vi "Project Wizard.vi"() -> ()   [LabVIEW 2021]
uses:
  Control/Tab Control.ctl
  Control/Available Sample List.ctl
  Control/Available List Item.ctl
  <vilib>/myRIO/Common/Instrument Driver Framework/Utilities/xctls/myRIO Choice Button/myRIO Choice Button.xctl
  Control/Shared Values.ctl
  Control/Item List.ctl
  Control/Item Info.ctl
  Control/Answers.ctl
  Control/Question.ctl
  Control/Answer.ctl
  Control/FP Values.ctl
  Control/Navigation Control.ctl
  Control/States.ctl
  <resource>/dialog/NewProjectWizard/SpecPage/Base/BaseSpecPage.lvclass
  <vilib>/event_ctls.llb/eventvkey.ctl
  <resource>/dialog/NewProjectWizard/MetaDataObj/MetaDataObj.lvclass/MetaDataObj.ctl
  <vilib>/Utility/miscctls.llb/LVRectTypeDef.ctl
  <resource>/dialog/NewProjectWizard/Spec Page Interface.ctl
  <resource>/dialog/NewProjectWizard/MetaDataObj/Accessors/Read Project Root.vi
  <resource>/dialog/NewProjectWizard/MetaDataObj/Accessors/Read File Prefix.vi
  <resource>/dialog/NewProjectWizard/MetaDataObj/Accessors/Read Project Name.vi
  <resource>/dialog/NewProjectWizard/MetaDataObj/Accessors/Read Overlay Pixmap.vi
  <resource>/dialog/NewProjectWizard/MetaDataObj/Accessors/Write Project Root.vi
  <vilib>/Utility/cursorutil.llb/Set Cursor (Icon Pict).vi
  <vilib>/Utility/xml.llb/Read From XML File(string).vi
  <vilib>/Platform/browser.llb/Open URL in Default Browser (path).vi
  <resource>/dialog/NewProjectWizard/MetaDataObj/Accessors/Read Custom VI Path.vi
  <resource>/dialog/NewProjectWizard/MetaDataObj/Accessors/Read Project Path.vi
  SubVI/Wizard Global.vi
  <resource>/dialog/NewProjectWizard/MetaDataObj/Accessors/Read Title.vi
  <resource>/dialog/NewProjectWizard/MetaDataObj/MetaDataObj.lvclass
  <vilib>/LabVIEW Icon API/lv_icon/Classes/Icon/Icon.lvclass
  <resource>/dialog/NewProjectWizard/Loading Project Info/NI_NPW_Loading Project Info.lvlib
  <resource>/dialog/NewProjectWizard/Filters/NI_NPW_Filters.lvlib
  <resource>/dialog/lvconfig.llb/LV Config Read Pathlist.vi
  <resource>/dialog/NewProjectWizard/MetaDataObj/Convert To Child Class.vi
  <resource>/dialog/NewProjectWizard/Init Spec Page.vi
  <resource>/dialog/NewProjectWizard/Build Error String.vi
  SubVI/Tab Key Process.vi
  <resource>/dialog/NewProjectWizard/ValidateFilePath.vi
  <resource>/dialog/lvconfig.llb/LV Config Write Pathlist.vi
  <resource>/dialog/NewProjectWizard/Project Copying/CreateUserProject.vi
  <resource>/dialog/NewProjectWizard/Project Copying/NI_NPW_Project Copying.lvlib
  <vilib>/Utility/cursorutil.llb/Set Busy.vi
  <resource>/dialog/NewProjectWizard/Defer Panel Updates.vi
panel:
  in  "Tab Control":T1
  in  "Choice 2":bool(xcontrol)
  in  "Choice 1":bool(xcontrol)
  out "Question":string="What's your task?"
  out "Recommended sample":string
  out "Recommend":string="Recommended sample project: "
  out "Description":string
  out "Sample Pic 2":picture caption="Template Pic"
  in  "More Information":string="More Information"
  in  "Scrollbar":i32(c297)
  in  "Sample Project":T2={"List Item"={"Name"="", "Description"="", "More Info"="More Information"}, "List Item 2"={"Name"="", "Description"="", "More Info"="More Information"}, "List Item 3"={"Name"="", "Description"="", "More Info"="More Information"}, "List Item 4"={"Name"="", "Description"="", "More Info"="More Information"}, "List Item 5"={"Name"="", "Description"="", "More Info"="More Information"}}
  in  "Sample Highlight":picture
  in  "Category:":string(tree)="Connection 2"
  out "Sample Pic":picture
  out "Error Messages":string
  in  "Cancel":bool
  in  "Next":bool
  in  "Back":bool
  # "Sample Project:"
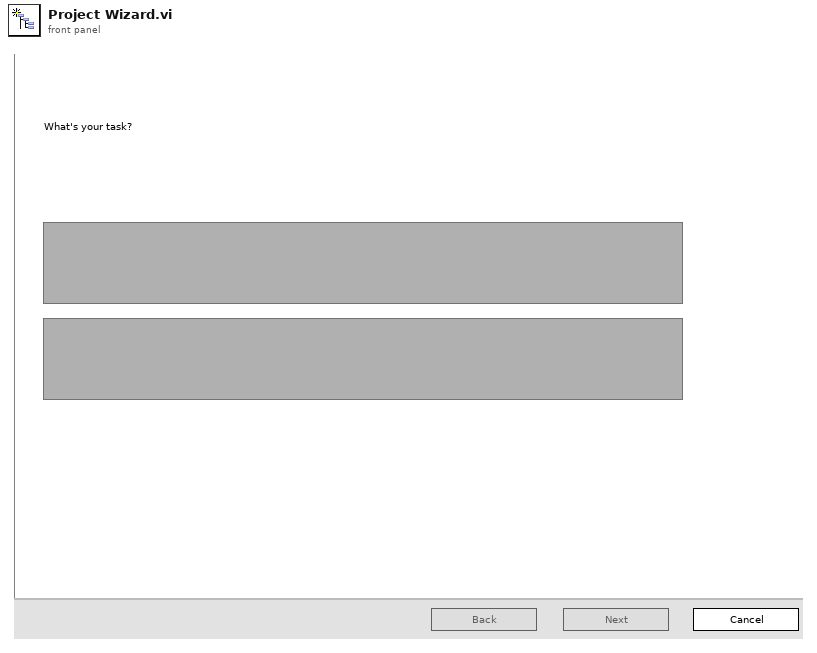
[diagram p1: front panel]
types:
  T1 = typedef "Tab Control.ctl" = enum32{"Start Page", "Recommend Sample", "Select Sample", "Configure Project"}
  T2 = typedef "Available Sample List.ctl" = cluster{"List Item":T3, "List Item 2":T3, "List Item 3":T3, "List Item 4":T3, "List Item 5":T3}
  T3 = typedef "Available List Item.ctl" = cluster{"Name":string, "Description":string, "More Info":string}
  T4 = typedef "States.ctl" = enum16{"Idle", "Initialize", "Parse Config Files", "Update Title", "Update Navigation", "Update Tab", "Load Question", "Load All Samples", "Update Sample Description", "Load Available Samples", "Cancel", "More Information", "Create Project", "Copy Project", "Update Warning", "Update Available Samples", "Select Available Sample", "Load Start Choice", "Show Recommended Sample", "Init Spec Page", "Insert Spec Page", "Stop Spec Page", "Set Control Font", "Focus Previous Selection"}
  T5 = typedef "FP Values.ctl" = cluster{"Title Index":i32, "Navigation Status":T6, "Selected Question":i32, "Selected Sample":i32, "Warning":string, "Sample Filter":string, "Available Items":T3[], "Scrollbar Value":i32, "Question":string, "Result":string, "Answers":T7, "Show Guidance":bool, "Tab Control":T1, "Previous Selection":T7}
  T6 = typedef "Navigation Control.ctl" = enum16{"Back Disable&Next", "Back Enable&Finish Disable", "Back Enable&Next", "Back Diable&Finish", "Back Enable&Finish", "Back Enable&Next Disable", "Back Disable&Next Disable"}
  T7 = typedef "Answers.ctl" = enum16{"Choice 1", "Choice 2"}
  T8 = typedef "Shared Values.ctl" = cluster{"Item List":T9, "Have Next Page":bool, "Next Page\n Index":i32, "User changed folder":bool, "Question Selection":i32[], "Selected Choices":T7[], "Sample Item Names":string[], "Displayed Available Sample":T3[], "Question List":T11[], "CurPage Ctrl #1":refnum<vi>, "CurPage Ctrl #n":refnum<vi>, "User Project":refnum<vi>, "Spec Page Reference":refnum<vi>, "Current Choice Index":i32}
  T9 = typedef "Item List.ctl" = T10[]
  T10 = typedef "Item Info.ctl" = cluster{"Tag Name":string, "Text":string, "Parent Tag":string, "Children Tags":string[], "Description":string, "Pic Name":string, "Is Root":bool, "Is Leaf":bool, "Sample Folder Name":string, "Documentation Name":string}
  T11 = typedef "Question.ctl" = cluster{"Text":string, "Choice 1":T12, "Choice 2":T12}
  T12 = typedef "Answer.ctl" = cluster{"Text":string, "ReachSample":bool, "Sample":string, "NextQuestion":i32}
  T13 = typedef "eventvkey.ctl" = enum16{"ASCII", "Enter", "Return", "Shift", "Ctrl", "Alt", "Cmd", "Opt", "Caps", "NumLock", "Clear", "Break", "Up", "Down", "Left", "Right", "Insert", "Delete", "Home", "End", "PageUp", "PageDown", "Escape", "Help", "Pause", "ScrollLock", "F1", "F2", "F3", "F4", "F5", "F6", "F7", "F8", "F9", "F10", "F11", "F12", "F13", "F14", "F15", "F16", "F17", "F18", "F19", "F20", "F21", "F22", "F23", "F24", "Play", "VolumeUp", "VolumeDown", "Mute", "Two Byte Char"}
  T14 = typedef "LVRectTypeDef.ctl" = cluster{"Left":i16, "Top":i16, "Right":i16, "Bottom":i16}
  T15 = enum8{"Enabled", "Disabled", "Disabled and Grayed Out"}
  T16 = typedef "LVPositionTypeDef.ctl" = cluster{"Left":i32, "Top":i32}
  T17 = typedef "Spec Page Interface.ctl" = cluster{"\"Tab Forward To\" Refnum":refnum<vi>, "\"Tab Backward To\" Refnum":refnum<vi>, "Errors":refnum<user-event>, "Quit":refnum<user-event>}
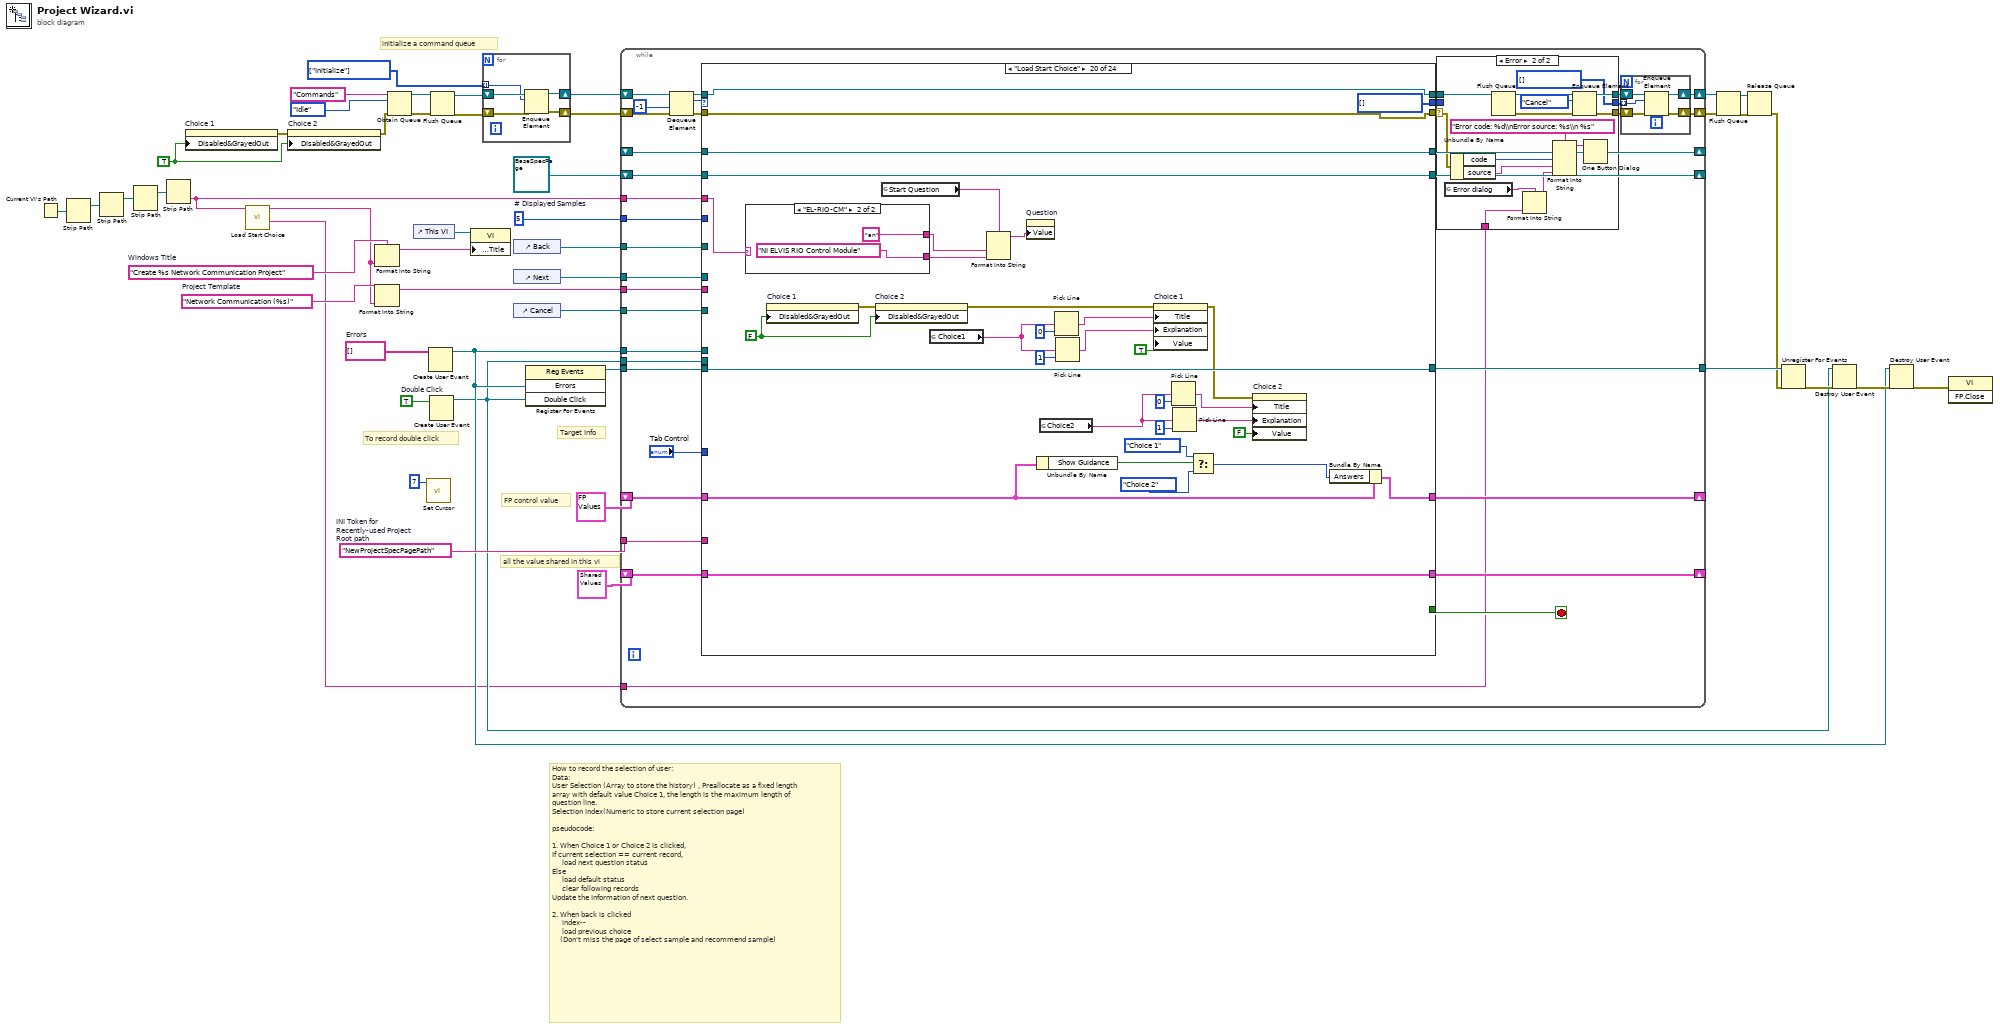
[diagram p0: block diagram]
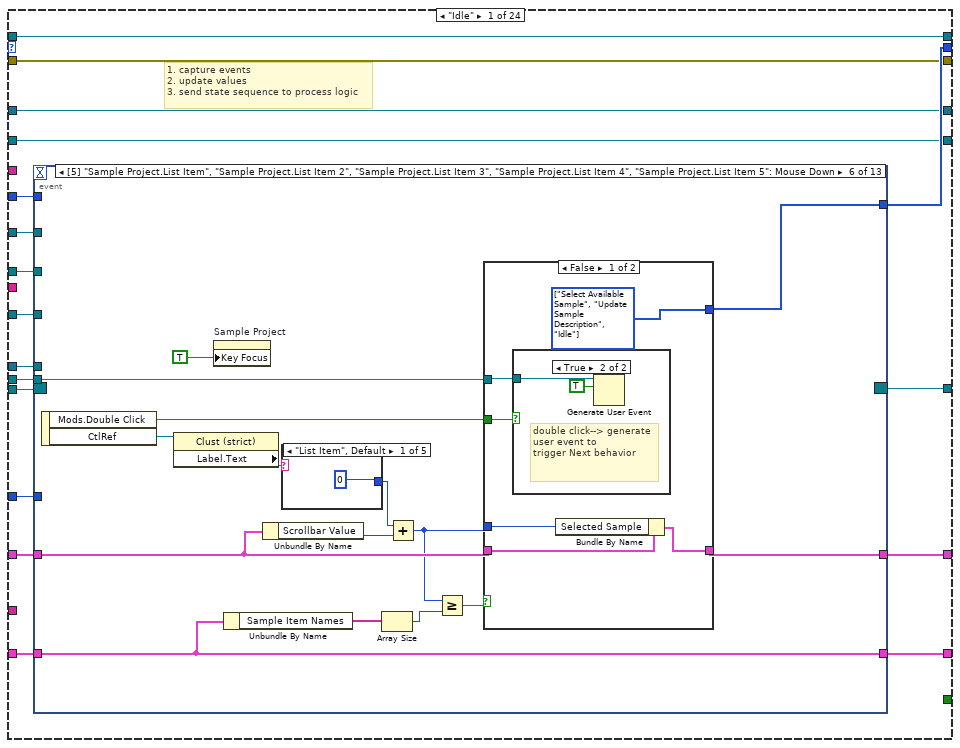
[diagram p3: hidden frame]
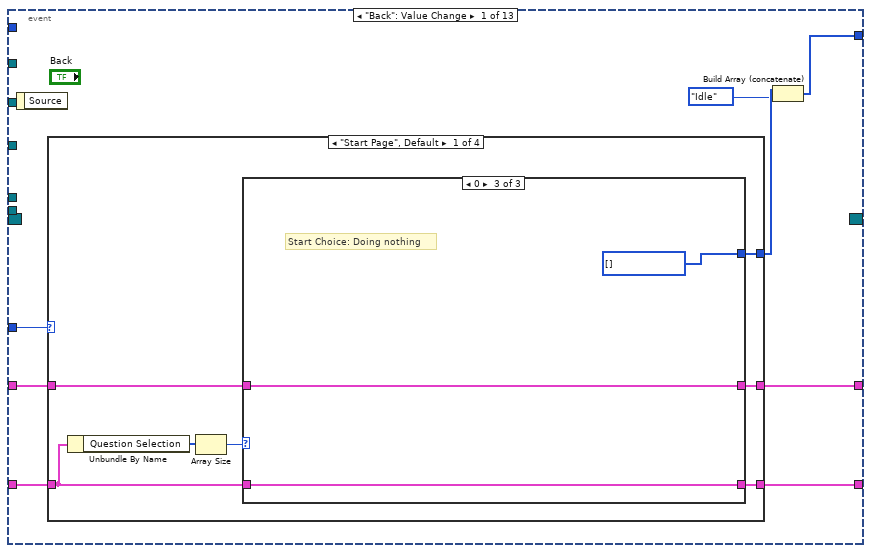
[diagram p4: hidden frame]
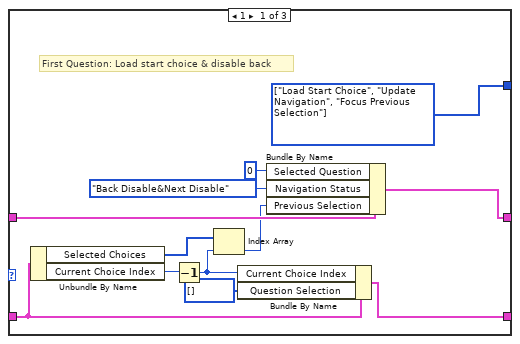
[diagram p5: hidden frame]
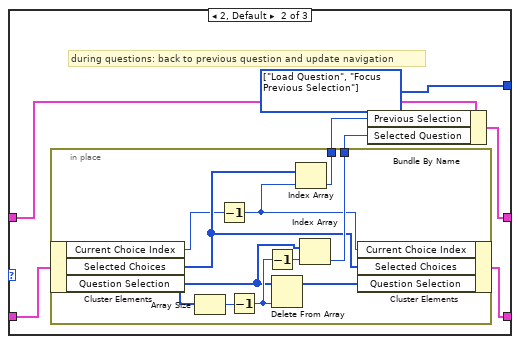
[diagram p6: hidden frame]
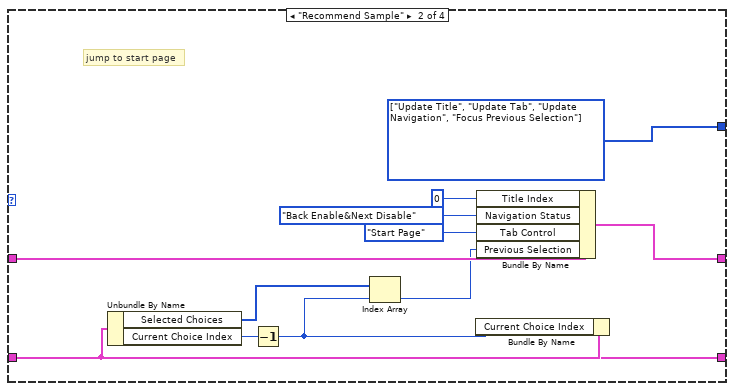
[diagram p7: hidden frame]
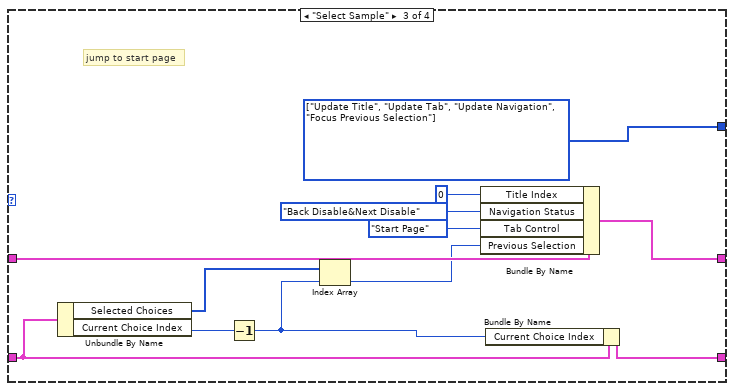
[diagram p8: hidden frame]
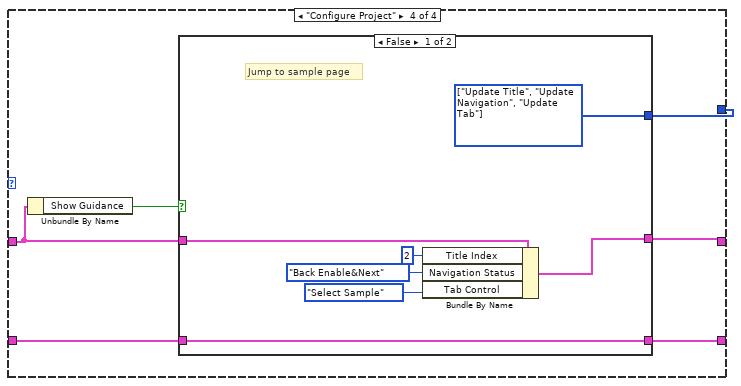
[diagram p9: hidden frame]
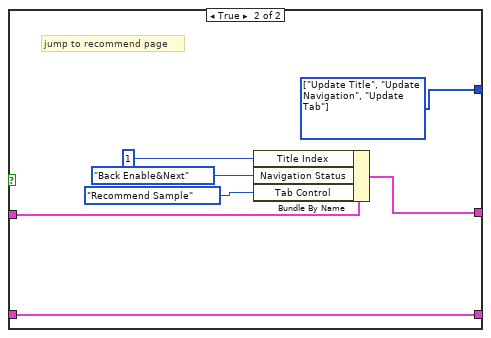
[diagram p10: hidden frame]
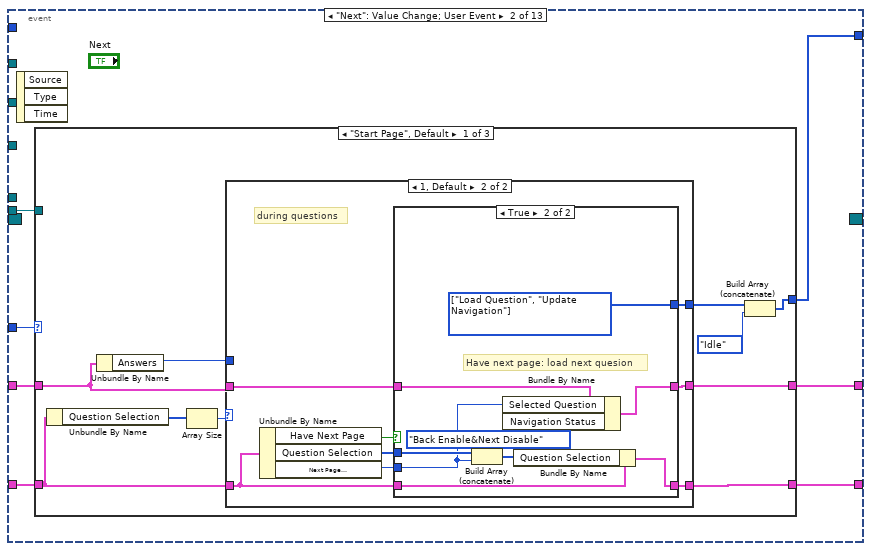
[diagram p11: hidden frame]
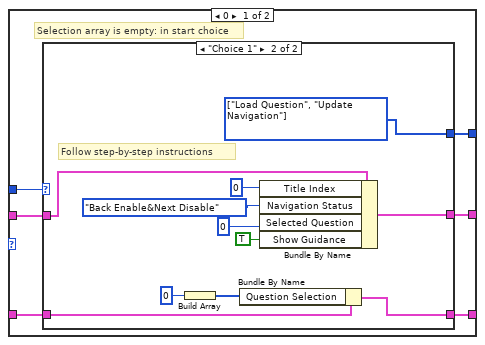
[diagram p12: hidden frame]
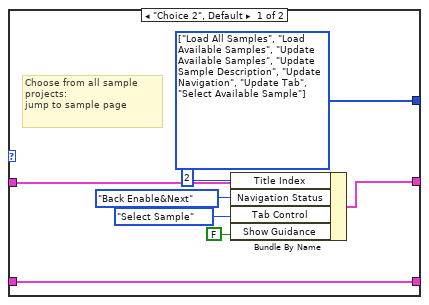
[diagram p13: hidden frame]
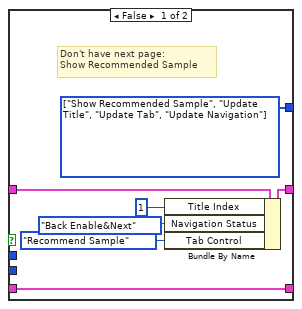
[diagram p14: hidden frame]
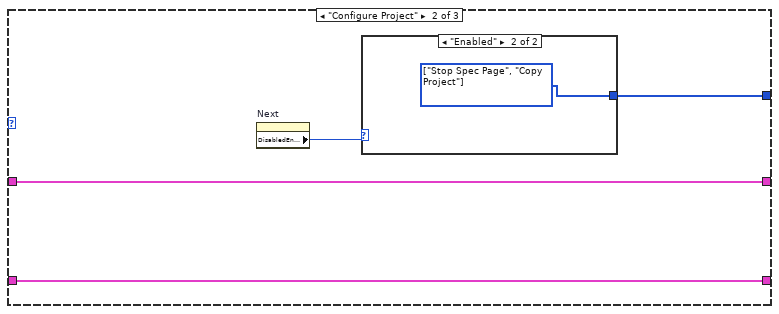
[diagram p15: hidden frame]
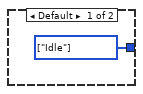
[diagram p16: hidden frame]
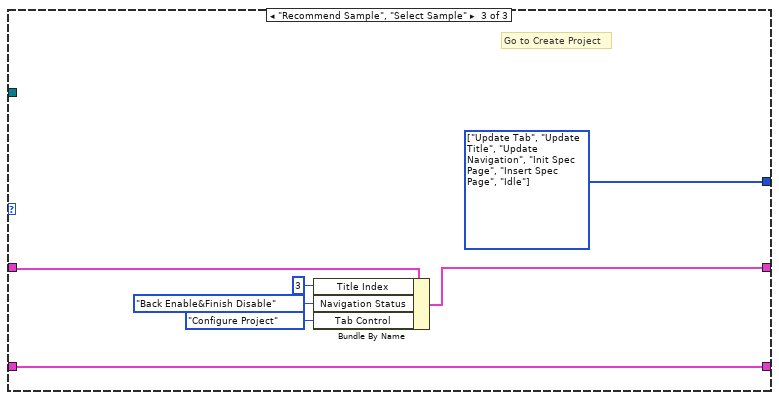
[diagram p17: hidden frame]
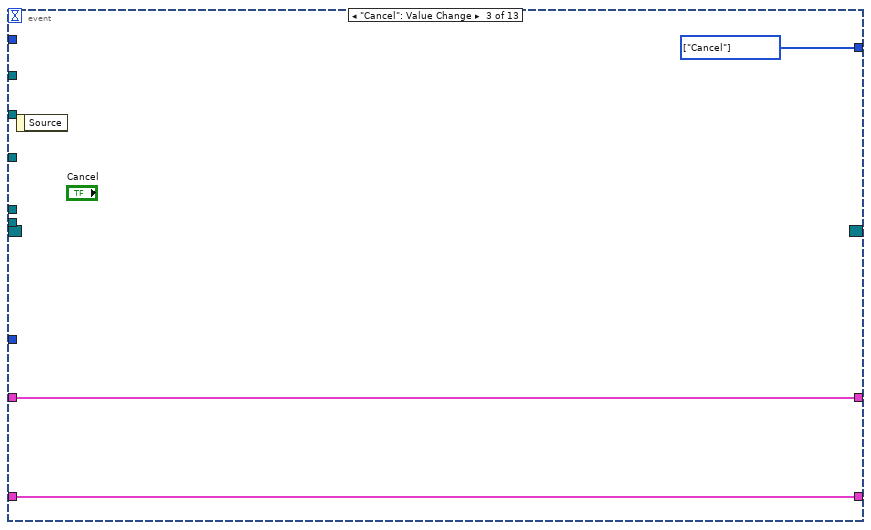
[diagram p18: hidden frame]
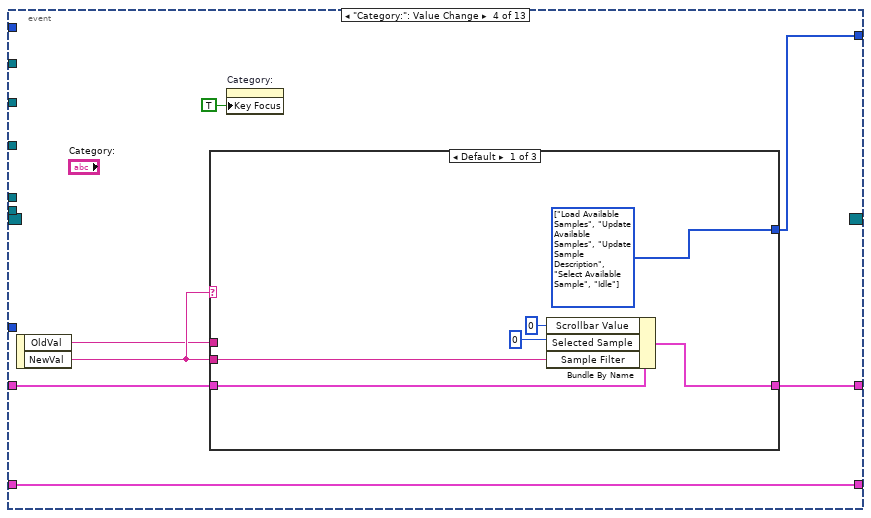
[diagram p19: hidden frame]
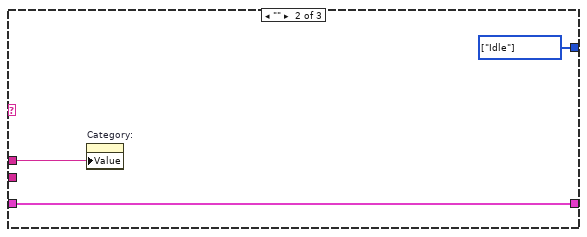
[diagram p20: hidden frame]
diagram:
  w11 = "Create %s Network Communication Project"  # Windows Title
  w18 = TRUE ("Disabled&GrayedOut")
  w25 = TRUE  # Double Click
  w27 = 5  # # Displayed Samples
  w12 = "Network Communication (%s)"  # Project Template
  w29 = "NewProjectSpecPagePath"  # INI Token for Recently-used Project Root path
  w36 = string[] []  # Errors
  w37 = T4[] [enum."Initialize"] items=["Idle", "Initialize", "Parse Config Files", "Update Title", "Update Navigation", "Update Tab", "Load Question", "Load All Samples", "Update Sample Description", "Load Available Samples", "Cancel", "More Information", "Create Project", "Copy Project", "Update Warning", "Update Available Samples", "Select Available Sample", "Load Start Choice", "Show Recommended Sample", "Init Spec Page", "Insert Spec Page", "Stop Spec Page", "Set Control Font", "Focus Previous Selection"]
  # "How to record the selection of user:\nData: \nUser Selection (Array to store the history) , Preallocate as a fixed length array with default value Choice 1, the length is the maximum length of question line.\nSelection Index(Numeric to store current selection page)\n\npseudocode:\n \n1. When Choice 1 or Choice 2 is clicked,\nIf current selection == current record,\n     load next question status\nElse\n     load default status\n     clear following records\nUpdate the Information of next question.\n\n2. When back is clicked    \n     index--\n     load previous choice\n    (Don't miss the page of select sample and recommend sample)"
  # "To record double click"
  # "Target Info"
  # "FP control value"
  # "all the value shared in this vi"
  # "initialize a command queue"
  n1 = Current VI's Path() -> (path=w17:path)
  n2 = Strip Path(path=w17) -> (stripped path=w16:path)  [unwired: 1 out]
  n3 = Strip Path(path=w16) -> (stripped path=w15:path)  [unwired: 1 out]
  n4 = Strip Path(path=w15) -> (stripped path=w14:path)  [unwired: 1 out]
  n5 = Strip Path(path=w14) -> (name=w2:string)  [unwired: 1 out]
  n6 = property on="Choice 1" class="myRIO Choice Button (strict)"("Disabled&GrayedOut"=w18) -> (error out=w20:errorcluster)  [unwired: 2 in, 1 out]
  n7 = call "Load Start Choice.vi"("Folder Name In"=w2) -> ("Toolkit Name"=w1:string, "Target Name"=w3:string)  [unwired: 9 in]
  n8 = property on="Choice 2" class="myRIO Choice Button (strict)"(error in=w20, "Disabled&GrayedOut"=w18) -> (error out=w19:errorcluster)  [unwired: 1 in, 1 out]
  n9 = Format Into String(format string=w11, w3) -> (resulting string=w9:string)  [unwired: 2 in, 1 out]
  n10 = Format Into String(format string=w12, w3) -> (resulting string=w13:string)  [unwired: 2 in, 1 out]
  n11 = Obtain Queue(name (unnamed)="Commands", element data type=States."Idle" ("States"), error in (no error)=w19) -> (queue out=w44:refnum<queue>, error out=w45:errorcluster)  [unwired: 2 in, 1 out]
  n12 = control-ref of="This VI"() -> (w10:refnum<vi>)
  n13 = call-poly <vilib>:"Set Cursor.vi"("icon"=u16 7) -> ()  [unwired: 9 in, 2 out]
  n14 = Create User Event(user event datatype=w36) -> (user event=w6:refnum<user-event>)  [unwired: 1 in, 1 out]
  n15 = Create User Event(user event datatype=w25) -> (user event=w5:refnum<user-event>)  [unwired: 1 in, 1 out]
  n16 = Flush Queue(queue=w44, error in (no error)=w45) -> (queue out=w43:refnum<queue>, error out=w42:errorcluster)  [unwired: 1 out]
  n17 = property class="VI"(reference=w10, "Front Panel.Title"=w9) -> ()  [unwired: 1 in, 2 out]
  n18 = for {
    shift-right: [w51] -> w47
    shift-left: w43 -> [w52]
    shift-right: [w49] -> w41
    shift-left: w42 -> [w50]
    tunnel: w37 -> [w48] mode=indexing
    n19 = Enqueue Element(queue=w52, element=w48, error in (no error)=w50) -> (queue out=w51:refnum<queue>, error out=w49:errorcluster)  [unwired: 1 in, 1 out]
  }
  n20 = control-ref of="Back"() -> (w35:refnum<vi>)
  n21 = control-ref of="Next"() -> (w26:refnum<vi>)
  n22 = control-ref of="Cancel"() -> (w33:refnum<vi>)
  n23 = register-events(w6, w5) -> (reference out=w34:refnum<event-registration>)  [unwired: 2 in, 1 out]
  n24 = while {
    shift-right: [w84] -> w24
    shift-left: w47 -> [w77]
    shift-right: [w81] -> w21
    shift-left: w41 -> [w85]
    shift-right: [w82] -> _
    shift-left: T8 {"Item List"=[], "Have Next Page"=FALSE, "Next Page\n Index"=0, "User changed folder"=FALSE, "Question Selection"=[], "Selected Choices"=[], "Sample Item Names"=[], "Displayed Available Sample"=[], "Question List"=[], "CurPage Ctrl #1"=refnum, "CurPage Ctrl #n"=refnum, "User Project"=refnum, "Spec Page Reference"=refnum, "Current Choice Index"=0} ("Shared Values") -> [w55]
    shift-right: [w78] -> _
    shift-left: T5 {"Title Index"=0, "Navigation Status"=enum."Back Disable&Next", "Selected Question"=0, "Selected Sample"=0, "Warning"="", "Sample Filter"="", "Available Items"=[], "Scrollbar Value"=0, "Question"="", "Result"="", "Answers"=enum."Choice 1", "Show Guidance"=FALSE, "Tab Control"=enum."Start Page", "Previous Selection"=enum."Choice 1"} ("FP Values") -> [w76]
    shift-right: [w75] -> _
    shift-left: _ -> [w74]
    tunnel: w26 -> [w73]
    tunnel: w35 -> [w72]
    tunnel: w6 -> [w70]
    tunnel: w34 -> [w69]
    tunnel: w33 -> [w71]
    tunnel: [w68] -> w31
    tunnel: w29 -> [w61]
    shift-right: [w59] -> _
    shift-left: refnum<class "BaseSpecPage.lvclass"> refnum ("BaseSpecPage out") -> [w60]
    tunnel: w13 -> [w58]
    tunnel: w27 -> [w57]
    tunnel: w5 -> [w56]
    tunnel: w2 -> [w54]
    tunnel: w1 -> [w53]
    stop <- w83 stop-if-true
    n25 = Dequeue Element(queue=w77, timeout in ms (-1)=-1, error in (no error)=w85) -> (queue out=w86:refnum<queue>, element=w79:T4, error out=w87:errorcluster)  [unwired: 1 out]
    n26 = case shown="\"Load Start Choice\"" w79 {
      tunnel: w87 -> [w122 w556 w577 w609 w644 w655 w664 w691 w705 w713 w727 w761 w794 w812 w850 w869 w915 w954 w965 w1049 w1058 w1074 w1124 w1154]
      tunnel: w86 -> [w128 w565 w578 w613 w642 w654 w662 w694 w706 w720 w735 w762 w804 w836 w867 w890 w913 w955 w975 w1050 w1068 w1095 w1143 w1161]
      tunnel: [w128 w565 w578 w613 w642 w654 w662 w694 w706 w720 w735 w762 w804 w836 w867 w890 w913 w955 w975 w1050 w1068 w1095 w1143 w1161] -> w63
      tunnel: [w122 w556 w577 w608 w644 w655 w664 w691 w705 w712 w734 w751 w792 w811 w849 w872 w915 w954 w964 w1049 w1057 w1073 w1121 w1153] -> w67
      tunnel: [_ _ _ _ _ _ _ _ _ _ _ _ TRUE _ _ _ _ _ _ _ _ _ _ _] -> w83
      tunnel: "Tab Control" -> [w129 _ _ _ _ _ _ _ _ _ _ _ _ _ _ _ _ _ _ _ _ _ _ _]
      tunnel: [w124 w564 w571 w604 w635 w645 w656 w675 w696 w708 w722 w744 w789 w833 w847 w873 w907 w941 w963 w1039 w1056 w1072 w1107 w1148] -> w66
      tunnel: w55 -> [w127 w553 w576 w612 w643 w653 w663 w688 w704 w716 w733 w760 w795 w827 w862 w875 w914 w952 w974 w1048 w1067 w1094 w1129 w1149]
      tunnel: [w126 w550 w576 w611 w643 w653 w663 w687 w704 w716 w733 w759 w795 w827 w862 w874 w914 w952 w974 w1048 w1067 w1094 w1136 w1149] -> w82
      tunnel: w76 -> [w125 w559 w575 w610 w641 w651 w660 w681 w700 w719 w726 w753 w796 w828 w866 w889 w912 w953 w973 w1044 w1066 w1093 w1130 w1160]
      tunnel: [w123 w560 w575 w610 w641 w651 w660 w680 w700 w718 w726 w752 w796 w828 w866 w889 w912 w953 w973 w1043 w1066 w1093 w1130 w1160] -> w78
      tunnel: [w121 w555 w574 w607 w638 w650 w659 w678 w703 w711 w725 w741 w802 w823 w864 w876 w911 w951 w969 w1042 w1061 w1084 w1114 w1155] -> w75
      tunnel: w74 -> [w121 w555 w574 w607 w638 w650 w659 w678 w703 w711 w725 w741 w802 w823 w864 w870 w911 w951 w969 w1042 w1061 _ w1115 w1156]
      tunnel: w73 -> [w118 _ _ _ _ w648 _ _ _ _ _ _ _ _ _ _ _ _ _ _ _ _ _ _]
      tunnel: w72 -> [w119 _ _ _ _ w649 _ _ _ _ _ _ _ _ _ _ _ _ _ _ _ _ w1140 _]
      tunnel: w71 -> [w117 _ _ _ _ _ _ _ _ _ _ _ _ _ _ _ _ _ _ _ _ _ w1139 _]
      tunnel: w70 -> [w115 _ _ _ _ _ _ _ _ _ _ _ _ _ _ _ _ _ _ _ _ _ w1138 _]
      tunnel: w69 -> [w120 w554 w573 w606 w637 w647 w658 w677 w702 w710 w724 w740 w801 w835 w865 w888 w910 w950 w968 w1041 w1060 w1083 w1134 w1159]
      tunnel: [w116 w554 w573 w606 w637 w647 w658 w677 w702 w710 w724 w740 w801 w835 w865 w888 w910 w950 w968 w1041 w1060 w1083 w1134 w1159] -> w68
      tunnel: w61 -> [_ _ _ _ _ _ _ _ _ _ _ _ _ _ _ w871 _ _ _ _ _ w1082 _ _]
      tunnel: w60 -> [w114 w552 w572 w605 w636 w646 w657 w676 w701 w709 w723 w739 w797 w834 w848 w868 w908 w949 w967 w1040 w1059 w1081 w1118 w1152]
      tunnel: [w114 w552 w572 w605 w636 w646 w657 w676 w701 w709 w723 w739 w797 w834 w848 w868 w908 w949 w967 w1040 w1059 w1081 w1117 w1151] -> w59
      tunnel: w58 -> [_ _ _ _ _ _ _ _ _ _ _ _ _ _ _ _ _ _ _ _ _ w1077 _ _]
      tunnel: w57 -> [w113 _ _ _ _ _ _ _ _ _ _ w737 _ _ _ _ _ _ _ _ _ _ _ _]
      tunnel: w56 -> [w112 _ _ _ _ _ _ _ _ _ _ _ _ _ _ _ _ _ _ _ _ _ _ _]
      tunnel: w54 -> [_ _ _ w603 _ _ _ _ _ _ w721 w736 _ _ _ _ _ _ _ w1020 w1055 _ _ _]
      frame "Idle" {
        # "1. capture events\n2. update values \n3. send state sequence to process logic"
        n27 = event shown="[5] \"Sample Project.List Item\", \"Sample Project.List Item 2\", \"Sample Project.List Item 3\", \"Sample Project.List Item 4\", \"Sample Project.List Item 5\": Mouse Down" {
          selector: w120 -> [_ _ _ _ _ _ _ _ _ _ _ _ _]
          dyn-events: [_ _ _ _ _ _ _ _ _ _ _ _ _] -> w116
          timeout: _ -> [_ _ _ _ _ _ _ _ _ _ _ _ _]
          tunnel: w129 -> [w137 w227 _ _ _ _ _ _ _ _ _ w427 _]
          tunnel: w127 -> [w133 w225 w302 w307 w330 w359 w378 w396 w402 w405 w413 w431 w503]
          tunnel: [w135 w224 w302 w307 w329 w359 w378 w396 w402 w405 w413 w431 w502] -> w126
          tunnel: w125 -> [w134 w223 w300 w309 w326 w355 w379 w395 w401 w404 w409 w421 w494]
          tunnel: [w136 w226 w300 w308 w325 w361 w379 w395 w401 w404 w408 w420 w493] -> w123
          tunnel: [w130 w221 w301 w304 w327 w347 w377 w392 w398 w403 w412 w418 w501] -> w124
          tunnel: w119 -> [_ _ _ _ _ _ _ _ _ _ _ w435 _]
          tunnel: w118 -> [_ _ _ _ _ _ _ _ _ _ _ w434 _]
          tunnel: w117 -> [_ _ _ _ _ _ _ _ _ _ _ w432 _]
          tunnel: w115 -> [_ _ _ _ _ _ _ _ _ _ _ _ _]
          tunnel: w113 -> [_ _ _ _ _ _ _ _ _ _ _ w423 _]
          tunnel: w112 -> [_ w222 _ _ _ w348 _ _ _ _ _ _ w505]
          event "Back": Value Change {
            n28 = event-data() -> ()  [unwired: 1 in, 1 out]
            n29 = case shown="\"Start Page\", Default" w137 {
              tunnel: [w138 w187 w199 w205] -> w132
              tunnel: w134 -> [w142 w188 w200 w202]
              tunnel: w133 -> [w141 w181 w193 w204]
              tunnel: [w139 w180 w192 w203] -> w135
              tunnel: [w140 w186 w198 w206] -> w136
              frame "Start Page", Default {
                n30 = Unbundle By Name(w141) -> ("Question Selection"=w144:i32[])
                n31 = Array Size(array=w144) -> (size(s)=w143:i32)
                n32 = case shown="0" w143 {
                  tunnel: w142 -> [w155 w161 w176]
                  tunnel: w141 -> [w149 w163 w175]
                  tunnel: [w154 w159 w176] -> w140
                  tunnel: [w151 w162 w175] -> w139
                  tunnel: [w156 w158 w174] -> w138
                  frame 1 {
                    w156 = T4[] [enum."Load Start Choice", enum."Update Navigation", enum."Focus Previous Selection"] items=["Idle", "Initialize", "Parse Config Files", "Update Title", "Update Navigation", "Update Tab", "Load Question", "Load All Samples", "Update Sample Description", "Load Available Samples", "Cancel", "More Information", "Create Project", "Copy Project", "Update Warning", "Update Available Samples", "Select Available Sample", "Load Start Choice", "Show Recommended Sample", "Init Spec Page", "Insert Spec Page", "Stop Spec Page", "Set Control Font", "Focus Previous Selection"]
                    # "First Question: Load start choice & disable back"
                    n33 = Unbundle By Name(w149) -> ("Selected Choices"=w146:T7[], "Current Choice Index"=w148:i32)
                    n34 = Decrement(x=w148) -> (x-1=w147:i32)
                    n35 = Index Array(array=w146, index=w147) -> (element=w145:T7)
                    n36 = Bundle By Name(cluster=w149, "Current Choice Index"=w147, "Question Selection"=i32[] []) -> (w151:T8)
                    n37 = Bundle By Name(cluster=w155, "Selected Question"=0 ("Selected Guidance"), "Navigation Status"=Navigation_Control."Back Disable&Next Disable", "Previous Selection"=w145) -> (w154:T5)
                  }
                  frame 2, Default {
                    w158 = T4[] [enum."Load Question", enum."Focus Previous Selection"] items=["Idle", "Initialize", "Parse Config Files", "Update Title", "Update Navigation", "Update Tab", "Load Question", "Load All Samples", "Update Sample Description", "Load Available Samples", "Cancel", "More Information", "Create Project", "Copy Project", "Update Warning", "Update Available Samples", "Select Available Sample", "Load Start Choice", "Show Recommended Sample", "Init Spec Page", "Insert Spec Page", "Stop Spec Page", "Set Control Font", "Focus Previous Selection"]
                    # "during questions: back to previous question and update navigation"
                    n38 = in-place {
                      in-place-border: [w168] -> w160
                      in-place-border: [w167] -> w157
                      n39 = in-place-cluster #1(w163) -> ("Current Choice Index"=w165:i32, "Selected Choices"=w166:T7[], "Question Selection"=w170:i32[])
                      n40 = Array Size(array=w170) -> (size(s)=w173:i32)
                      n41 = Decrement(x=w165) -> (x-1=w164:i32)
                      n42 = Decrement(x=w173) -> (x-1=w171:i32)
                      n43 = Decrement(x=w171) -> (x-1=w169:i32)
                      n44 = Delete From Array(array=w170, index=w171) -> (array with subset deleted=w172:i32[])  [unwired: 1 in, 1 out]
                      n45 = Index Array(array=w166, index=w164) -> (element=w167:T7)
                      n46 = Index Array(array=w170, index=w169) -> (element=w168:i32)
                      n47 = in-place-cluster #1("Current Choice Index"=w164, "Selected Choices"=w166, "Question Selection"=w172) -> (w162:T8)
                    }
                    n48 = Bundle By Name(cluster=w161, "Previous Selection"=w157, "Selected Question"=w160) -> (w159:T5)
                  }
                  frame 0 {
                    w174 = T4[] [] items=["Idle", "Initialize", "Parse Config Files", "Update Title", "Update Navigation", "Update Tab", "Load Question", "Load All Samples", "Update Sample Description", "Load Available Samples", "Cancel", "More Information", "Create Project", "Copy Project", "Update Warning", "Update Available Samples", "Select Available Sample", "Load Start Choice", "Show Recommended Sample", "Init Spec Page", "Insert Spec Page", "Stop Spec Page", "Set Control Font", "Focus Previous Selection"]
                    # "Start Choice: Doing nothing"
                  }
                }
              }
              frame "Recommend Sample" {
                w187 = T4[] [enum."Update Title", enum."Update Tab", enum."Update Navigation", enum."Focus Previous Selection"] items=["Idle", "Initialize", "Parse Config Files", "Update Title", "Update Navigation", "Update Tab", "Load Question", "Load All Samples", "Update Sample Description", "Load Available Samples", "Cancel", "More Information", "Create Project", "Copy Project", "Update Warning", "Update Available Samples", "Select Available Sample", "Load Start Choice", "Show Recommended Sample", "Init Spec Page", "Insert Spec Page", "Stop Spec Page", "Set Control Font", "Focus Previous Selection"]
                # "jump to start page"
                n49 = Unbundle By Name(w181) -> ("Selected Choices"=w182:T7[], "Current Choice Index"=w178:i32)
                n50 = Decrement(x=w178) -> (x-1=w177:i32)
                n51 = Index Array(array=w182, index=w177) -> (element=w179:T7)
                n52 = Bundle By Name(cluster=w181, "Current Choice Index"=w177) -> (w180:T8)
                n53 = Bundle By Name(cluster=w188, "Title Index"=0, "Navigation Status"=Navigation_Control."Back Enable&Next Disable", "Tab Control"=Tab_Control."Start Page", "Previous Selection"=w179) -> (w186:T5)
              }
              frame "Select Sample" {
                w199 = T4[] [enum."Update Title", enum."Update Tab", enum."Update Navigation", enum."Focus Previous Selection"] items=["Idle", "Initialize", "Parse Config Files", "Update Title", "Update Navigation", "Update Tab", "Load Question", "Load All Samples", "Update Sample Description", "Load Available Samples", "Cancel", "More Information", "Create Project", "Copy Project", "Update Warning", "Update Available Samples", "Select Available Sample", "Load Start Choice", "Show Recommended Sample", "Init Spec Page", "Insert Spec Page", "Stop Spec Page", "Set Control Font", "Focus Previous Selection"]
                # "jump to start page"
                n54 = Unbundle By Name(w193) -> ("Selected Choices"=w194:T7[], "Current Choice Index"=w191:i32)
                n55 = Decrement(x=w191) -> (x-1=w189:i32)
                n56 = Index Array(array=w194, index=w189) -> (element=w190:T7)
                n57 = Bundle By Name(cluster=w200, "Title Index"=0, "Navigation Status"=Navigation_Control."Back Disable&Next Disable", "Tab Control"=Tab_Control."Start Page", "Previous Selection"=w190) -> (w198:T5)
                n58 = Bundle By Name(cluster=w193, "Current Choice Index"=w189) -> (w192:T8)
              }
              frame "Configure Project" {
                n59 = Unbundle By Name(w202) -> ("Show Guidance"=w201:bool)
                n60 = case shown="False" w201 {
                  tunnel: [w210 w216] -> w206
                  tunnel: w202 -> [w209 w217]
                  tunnel: [w208 w215] -> w205
                  tunnel: w204 -> [w207 w214]
                  tunnel: [w207 w214] -> w203
                  frame False {
                    w208 = T4[] [enum."Update Title", enum."Update Navigation", enum."Update Tab"] items=["Idle", "Initialize", "Parse Config Files", "Update Title", "Update Navigation", "Update Tab", "Load Question", "Load All Samples", "Update Sample Description", "Load Available Samples", "Cancel", "More Information", "Create Project", "Copy Project", "Update Warning", "Update Available Samples", "Select Available Sample", "Load Start Choice", "Show Recommended Sample", "Init Spec Page", "Insert Spec Page", "Stop Spec Page", "Set Control Font", "Focus Previous Selection"]
                    # "Jump to sample page"
                    n61 = Bundle By Name(cluster=w209, "Title Index"=2, "Navigation Status"=Navigation_Control."Back Enable&Next", "Tab Control"=Tab_Control."Select Sample") -> (w210:T5)
                  }
                  frame True {
                    w215 = T4[] [enum."Update Title", enum."Update Navigation", enum."Update Tab"] items=["Idle", "Initialize", "Parse Config Files", "Update Title", "Update Navigation", "Update Tab", "Load Question", "Load All Samples", "Update Sample Description", "Load Available Samples", "Cancel", "More Information", "Create Project", "Copy Project", "Update Warning", "Update Available Samples", "Select Available Sample", "Load Start Choice", "Show Recommended Sample", "Init Spec Page", "Insert Spec Page", "Stop Spec Page", "Set Control Font", "Focus Previous Selection"]
                    # "jump to recommend page"
                    n62 = Bundle By Name(cluster=w217, "Title Index"=1 ("Page Index"), "Navigation Status"=Navigation_Control."Back Enable&Next", "Tab Control"=Tab_Control."Recommend Sample") -> (w216:T5)
                  }
                }
              }
            }
            n63 = Build Array (concatenate)(w132, States."Idle" ("States")) -> (w130:T4[])
          }
          event "Next": Value Change; User Event {
            n64 = event-data() -> ()  [unwired: 1 in, 3 out]
            n65 = case shown="\"Start Page\", Default" w227 {
              tunnel: w223 -> [w231 w288 w296]
              tunnel: [w237 w288 w294] -> w226
              tunnel: [w228 w290 w299] -> w221
              tunnel: w225 -> [w234 w289 w293]
              tunnel: [w235 w289 w293] -> w224
              tunnel: w222 -> [_ _ _]
              frame "Start Page", Default {
                n66 = Unbundle By Name(w234) -> ("Question Selection"=w233:i32[])
                n67 = Unbundle By Name(w231) -> ("Answers"=w230:T7)
                n68 = Array Size(array=w233) -> (size(s)=w232:i32)
                n69 = case shown="1, Default" w232 {
                  tunnel: [w243 w263] -> w237
                  tunnel: [w242 w270] -> w236
                  tunnel: [w241 w269] -> w235
                  tunnel: w234 -> [w240 w268]
                  tunnel: w231 -> [w239 w264]
                  tunnel: w230 -> [w238 _]
                  frame 0 {
                    # "Selection array is empty: in start choice"
                    n70 = case shown="\"Choice 1\"" w238 {
                      tunnel: w239 -> [w250 w262]
                      tunnel: [w251 w261] -> w243
                      tunnel: [w249 w258] -> w242
                      tunnel: w240 -> [w246 w256]
                      tunnel: [w246 w253] -> w241
                      frame "Choice 2", Default {
                        w249 = T4[] [enum."Load All Samples", enum."Load Available Samples", enum."Update Available Samples", enum."Update Sample Description", enum."Update Navigation", enum."Update Tab", enum."Select Available Sample"] items=["Idle", "Initialize", "Parse Config Files", "Update Title", "Update Navigation", "Update Tab", "Load Question", "Load All Samples", "Update Sample Description", "Load Available Samples", "Cancel", "More Information", "Create Project", "Copy Project", "Update Warning", "Update Available Samples", "Select Available Sample", "Load Start Choice", "Show Recommended Sample", "Init Spec Page", "Insert Spec Page", "Stop Spec Page", "Set Control Font", "Focus Previous Selection"]
                        # "Choose from all sample projects:\njump to sample page"
                        n71 = Bundle By Name(cluster=w250, "Title Index"=2 ("Page Index"), "Navigation Status"=Navigation_Control."Back Enable&Next", "Tab Control"=Tab_Control."Select Sample", "Show Guidance"=FALSE) -> (w251:T5)
                      }
                      frame "Choice 1" {
                        w258 = T4[] [enum."Load Question", enum."Update Navigation"] items=["Idle", "Initialize", "Parse Config Files", "Update Title", "Update Navigation", "Update Tab", "Load Question", "Load All Samples", "Update Sample Description", "Load Available Samples", "Cancel", "More Information", "Create Project", "Copy Project", "Update Warning", "Update Available Samples", "Select Available Sample", "Load Start Choice", "Show Recommended Sample", "Init Spec Page", "Insert Spec Page", "Stop Spec Page", "Set Control Font", "Focus Previous Selection"]
                        # "Follow step-by-step instructions"
                        n72 = Build Array(0) -> (w254:i32[])
                        n73 = Bundle By Name(cluster=w256, "Question Selection"=w254) -> (w253:T8)
                        n74 = Bundle By Name(cluster=w262, "Title Index"=0 ("Page Index"), "Navigation Status"=Navigation_Control."Back Enable&Next Disable", "Selected Question"=0 ("Selected Guidance"), "Show Guidance"=TRUE) -> (w261:T5)
                      }
                    }
                  }
                  frame 1, Default {
                    # "during questions"
                    n75 = Unbundle By Name(w268) -> ("Have Next Page"=w265:bool, "Question Selection"=w267:i32[], "Next Page\n Index"=w266:i32)
                    n76 = case shown="True" w265 {
                      tunnel: [w277 w286] -> w270
                      tunnel: [w276 w285] -> w269
                      tunnel: w268 -> [w276 w284]
                      tunnel: w267 -> [_ w283]
                      tunnel: w266 -> [_ w281]
                      tunnel: w264 -> [w272 w280]
                      tunnel: [w271 w279] -> w263
                      frame False {
                        w277 = T4[] [enum."Show Recommended Sample", enum."Update Title", enum."Update Tab", enum."Update Navigation"] items=["Idle", "Initialize", "Parse Config Files", "Update Title", "Update Navigation", "Update Tab", "Load Question", "Load All Samples", "Update Sample Description", "Load Available Samples", "Cancel", "More Information", "Create Project", "Copy Project", "Update Warning", "Update Available Samples", "Select Available Sample", "Load Start Choice", "Show Recommended Sample", "Init Spec Page", "Insert Spec Page", "Stop Spec Page", "Set Control Font", "Focus Previous Selection"]
                        # "Don't have next page:\nShow Recommended Sample"
                        n77 = Bundle By Name(cluster=w272, "Title Index"=1, "Navigation Status"=Navigation_Control."Back Enable&Next", "Tab Control"=Tab_Control."Recommend Sample") -> (w271:T5)
                      }
                      frame True {
                        w286 = T4[] [enum."Load Question", enum."Update Navigation"] items=["Idle", "Initialize", "Parse Config Files", "Update Title", "Update Navigation", "Update Tab", "Load Question", "Load All Samples", "Update Sample Description", "Load Available Samples", "Cancel", "More Information", "Create Project", "Copy Project", "Update Warning", "Update Available Samples", "Select Available Sample", "Load Start Choice", "Show Recommended Sample", "Init Spec Page", "Insert Spec Page", "Stop Spec Page", "Set Control Font", "Focus Previous Selection"]
                        # "Have next page: load next quesion"
                        n78 = Build Array (concatenate)(w283, w281) -> (w282:i32[])
                        n79 = Bundle By Name(cluster=w280, "Selected Question"=w281, "Navigation Status"=Navigation_Control."Back Enable&Next Disable") -> (w279:T5)
                        n80 = Bundle By Name(cluster=w284, "Question Selection"=w282) -> (w285:T8)
                      }
                    }
                  }
                }
                n81 = Build Array (concatenate)(w236, States."Idle" ("States")) -> (w228:T4[])
              }
              frame "Configure Project" {
                n82 = property on="Next" class="Bool"() -> ("DisabledEnum"=w287:T15)  [unwired: 2 in, 2 out]
                n83 = case shown="\"Enabled\"" w287 {
                  tunnel: [w291 w292] -> w290
                  frame Default {
                    w291 = T4[] [enum."Idle"] items=["Idle", "Initialize", "Parse Config Files", "Update Title", "Update Navigation", "Update Tab", "Load Question", "Load All Samples", "Update Sample Description", "Load Available Samples", "Cancel", "More Information", "Create Project", "Copy Project", "Update Warning", "Update Available Samples", "Select Available Sample", "Load Start Choice", "Show Recommended Sample", "Init Spec Page", "Insert Spec Page", "Stop Spec Page", "Set Control Font", "Focus Previous Selection"]
                  }
                  frame "Enabled" {
                    w292 = T4[] [enum."Stop Spec Page", enum."Copy Project"] items=["Idle", "Initialize", "Parse Config Files", "Update Title", "Update Navigation", "Update Tab", "Load Question", "Load All Samples", "Update Sample Description", "Load Available Samples", "Cancel", "More Information", "Create Project", "Copy Project", "Update Warning", "Update Available Samples", "Select Available Sample", "Load Start Choice", "Show Recommended Sample", "Init Spec Page", "Insert Spec Page", "Stop Spec Page", "Set Control Font", "Focus Previous Selection"]
                  }
                }
              }
              frame "Recommend Sample", "Select Sample" {
                w299 = T4[] [enum."Update Tab", enum."Update Title", enum."Update Navigation", enum."Init Spec Page", enum."Insert Spec Page", enum."Idle"] items=["Idle", "Initialize", "Parse Config Files", "Update Title", "Update Navigation", "Update Tab", "Load Question", "Load All Samples", "Update Sample Description", "Load Available Samples", "Cancel", "More Information", "Create Project", "Copy Project", "Update Warning", "Update Available Samples", "Select Available Sample", "Load Start Choice", "Show Recommended Sample", "Init Spec Page", "Insert Spec Page", "Stop Spec Page", "Set Control Font", "Focus Previous Selection"]
                # "Go to Create Project"
                n84 = Bundle By Name(cluster=w296, "Title Index"=3, "Navigation Status"=Navigation_Control."Back Enable&Finish Disable", "Tab Control"=Tab_Control."Configure Project") -> (w294:T5)
              }
            }
          }
          event "Cancel": Value Change {
            w301 = T4[] [enum."Cancel"] items=["Idle", "Initialize", "Parse Config Files", "Update Title", "Update Navigation", "Update Tab", "Load Question", "Load All Samples", "Update Sample Description", "Load Available Samples", "Cancel", "More Information", "Create Project", "Copy Project", "Update Warning", "Update Available Samples", "Select Available Sample", "Load Start Choice", "Show Recommended Sample", "Init Spec Page", "Insert Spec Page", "Stop Spec Page", "Set Control Font", "Focus Previous Selection"]
            n85 = event-data() -> ()  [unwired: 1 in, 1 out]
          }
          event "Category:": Value Change {
            n86 = event-data() -> ("OldVal"=w305:string, "NewVal"=w306:string)  [unwired: 1 in]
            n87 = case shown="Default" w306 {
              tunnel: w309 -> [w314 w318 w323]
              tunnel: [w313 w318 w322] -> w308
              tunnel: w306 -> [w312 _ _]
              tunnel: w305 -> [_ w316 _]
              tunnel: [w311 w317 w319] -> w304
              frame Default {
                w311 = T4[] [enum."Load Available Samples", enum."Update Available Samples", enum."Update Sample Description", enum."Select Available Sample", enum."Idle"] items=["Idle", "Initialize", "Parse Config Files", "Update Title", "Update Navigation", "Update Tab", "Load Question", "Load All Samples", "Update Sample Description", "Load Available Samples", "Cancel", "More Information", "Create Project", "Copy Project", "Update Warning", "Update Available Samples", "Select Available Sample", "Load Start Choice", "Show Recommended Sample", "Init Spec Page", "Insert Spec Page", "Stop Spec Page", "Set Control Font", "Focus Previous Selection"]
                n88 = Bundle By Name(cluster=w314, "Scrollbar Value"=0, "Selected Sample"=0, "Sample Filter"=w312) -> (w313:T5)
              }
              frame "" {
                w317 = T4[] [enum."Idle"] items=["Idle", "Initialize", "Parse Config Files", "Update Title", "Update Navigation", "Update Tab", "Load Question", "Load All Samples", "Update Sample Description", "Load Available Samples", "Cancel", "More Information", "Create Project", "Copy Project", "Update Warning", "Update Available Samples", "Select Available Sample", "Load Start Choice", "Show Recommended Sample", "Init Spec Page", "Insert Spec Page", "Stop Spec Page", "Set Control Font", "Focus Previous Selection"]
                n89 = property on="Category:" class="Tree (strict)"("Value"=w316) -> ()  [unwired: 2 in, 2 out]
              }
              frame "All Samples" {
                w319 = T4[] [enum."Load Available Samples", enum."Update Available Samples", enum."Update Sample Description", enum."Idle"] items=["Idle", "Initialize", "Parse Config Files", "Update Title", "Update Navigation", "Update Tab", "Load Question", "Load All Samples", "Update Sample Description", "Load Available Samples", "Cancel", "More Information", "Create Project", "Copy Project", "Update Warning", "Update Available Samples", "Select Available Sample", "Load Start Choice", "Show Recommended Sample", "Init Spec Page", "Insert Spec Page", "Stop Spec Page", "Set Control Font", "Focus Previous Selection"]
                n90 = Bundle By Name(cluster=w323, "Selected Sample"=0, "Sample Filter"="") -> (w322:T5)
              }
            }
            n91 = property on="Category:" class="Tree (strict)"("Key Focus"=TRUE) -> ()  [unwired: 2 in, 2 out]
          }
          event "Scrollbar": Value Change {
            w327 = T4[] [enum."Update Available Samples", enum."Select Available Sample", enum."Idle"] items=["Idle", "Initialize", "Parse Config Files", "Update Title", "Update Navigation", "Update Tab", "Load Question", "Load All Samples", "Update Sample Description", "Load Available Samples", "Cancel", "More Information", "Create Project", "Copy Project", "Update Warning", "Update Available Samples", "Select Available Sample", "Load Start Choice", "Show Recommended Sample", "Init Spec Page", "Insert Spec Page", "Stop Spec Page", "Set Control Font", "Focus Previous Selection"]
            n92 = event-data() -> ("NewVal"=w324:i32)  [unwired: 1 in]
            n93 = Unbundle By Name(w326) -> ("Available Items"=w331:T3[])
            n94 = Array Size(array=w331) -> (size(s)=w332:i32)
            n95 = for {
              N: 5 -> [_]
              tunnel: w331 -> [w342]
              tunnel: w324 -> [w341]
              tunnel: w332 -> [w336]
              tunnel: [w334] -> w328 mode=indexing
              i -> [w337]
              n96 = Add(x=w341, y=w337) -> (x+y=w339:i32)
              n97 = Increment(x=w336) -> (x+1=w335:i32)
              n98 = In Range and Coerce(upper limit=w335, x=w339, lower limit=0 ("y")) -> (In Range?=w340:bool)  [unwired: 1 out]
              n99 = case shown="False" w340 {
                tunnel: [T3 {"Name"="", "Description"="", "More Info"=""} ("List Item") w344] -> w334
                tunnel: w339 -> [_ w346]
                tunnel: w342 -> [_ w345]
                frame False {
                }
                frame True {
                  n100 = Index Array(array=w345, index=w346) -> (element=w344:T3)
                }
              }
            }
            n101 = Bundle By Name(cluster=w326, "Scrollbar Value"=w324) -> (w325:T5)
            n102 = Bundle By Name(cluster=w330, "Displayed Available Sample"=w328) -> (w329:T8)
          }
          event Mouse Down {
            n103 = event-data() -> ("Mods.Double Click"=w349:bool, "CtlRef"=w351:refnum<vi>)  [unwired: 1 in]
            n104 = property class="Clust (strict)"(reference=w351) -> ("Label.Text"=w360:string)  [unwired: 1 in, 2 out]
            n105 = property on="Sample Project" class="Clust (strict)"("Key Focus"=TRUE) -> ()  [unwired: 2 in, 2 out]
            n106 = Unbundle By Name(w359) -> ("Sample Item Names"=w358:string[])
            n107 = Unbundle By Name(w355) -> ("Scrollbar Value"=w353:i32)
            n108 = case shown="\"List Item\", Default" w360 {
              tunnel: [0 1 2 3 4] -> w354
              frame "List Item", Default {
              }
              frame "List Item 2" {
              }
              frame "List Item 3" {
              }
              frame "List Item 4" {
              }
              frame "List Item 5" {
              }
            }
            n109 = Array Size(array=w358) -> (size(s)=w357:i32)
            n110 = Add(x=w354, y=w353) -> (x+y=w352:i32)
            n111 = Greater Or Equal?(x=w352, y=w357) -> (x >= y?=w356:bool)
            n112 = case shown="False" w356 {
              tunnel: w355 -> [w367 w371]
              tunnel: [w366 w371] -> w361
              tunnel: w352 -> [w365 _]
              tunnel: w349 -> [w364 _]
              tunnel: w348 -> [w363 _]
              tunnel: [w362 w370] -> w347
              frame False {
                w362 = T4[] [enum."Select Available Sample", enum."Update Sample Description", enum."Idle"] items=["Idle", "Initialize", "Parse Config Files", "Update Title", "Update Navigation", "Update Tab", "Load Question", "Load All Samples", "Update Sample Description", "Load Available Samples", "Cancel", "More Information", "Create Project", "Copy Project", "Update Warning", "Update Available Samples", "Select Available Sample", "Load Start Choice", "Show Recommended Sample", "Init Spec Page", "Insert Spec Page", "Stop Spec Page", "Set Control Font", "Focus Previous Selection"]
                n113 = case shown="True" w364 {
                  tunnel: w363 -> [_ w368]
                  frame False {
                  }
                  frame True {
                    # "double click--> generate user event to \ntrigger Next behavior"
                    n114 = Generate User Event(user event=w368, event data cluster=TRUE ("event data")) -> ()  [unwired: 2 in, 2 out]
                  }
                }
                n115 = Bundle By Name(cluster=w367, "Selected Sample"=w365) -> (w366:T5)
              }
              frame True {
                w370 = T4[] [enum."Idle"] items=["Idle", "Initialize", "Parse Config Files", "Update Title", "Update Navigation", "Update Tab", "Load Question", "Load All Samples", "Update Sample Description", "Load Available Samples", "Cancel", "More Information", "Create Project", "Copy Project", "Update Warning", "Update Available Samples", "Select Available Sample", "Load Start Choice", "Show Recommended Sample", "Init Spec Page", "Insert Spec Page", "Stop Spec Page", "Set Control Font", "Focus Previous Selection"]
                # "select an empty item\n--> do nothing"
              }
            }
          }
          event Mouse Wheel {
            w377 = T4[] [enum."Idle"] items=["Idle", "Initialize", "Parse Config Files", "Update Title", "Update Navigation", "Update Tab", "Load Question", "Load All Samples", "Update Sample Description", "Load Available Samples", "Cancel", "More Information", "Create Project", "Copy Project", "Update Warning", "Update Available Samples", "Select Available Sample", "Load Start Choice", "Show Recommended Sample", "Init Spec Page", "Insert Spec Page", "Stop Spec Page", "Set Control Font", "Focus Previous Selection"]
            n116 = event-data() -> ("Delta"=w385:i32)  [unwired: 1 in, 1 out]
            n117 = property on="Scrollbar" class="Scroll (strict)"() -> ("Value"=w384:i32, "DocMax"=w383:dbl, "PageSize"=w382:dbl)  [unwired: 2 in, 2 out]
            n118 = Negate(x=w385) -> (-x=w387:i32)
            n119 = Subtract(x=w383, y=w382) -> (x-y=w386:dbl)
            n120 = Add(x=w384, y=w387) -> (x+y=w380:i32)
            n121 = Greater?(x=w380, y=w386) -> (0:w389:bool)
            n122 = Less Than 0?(x=w380) -> (x < 0?=w388:bool)
            n123 = Or(x=w388, y=w389) -> (x .or. y?=w381:bool)
            n124 = case shown="False" w381 {
              tunnel: w380 -> [_ w390]
              frame True {
              }
              frame False {
                n125 = property on="Scrollbar" class="Scroll (strict)"("Val(Sgnl)"=w390) -> ()  [unwired: 2 in, 2 out]
              }
            }
          }
          event "More Information": Mouse Enter {
            w392 = T4[] [enum."Idle"] items=["Idle", "Initialize", "Parse Config Files", "Update Title", "Update Navigation", "Update Tab", "Load Question", "Load All Samples", "Update Sample Description", "Load Available Samples", "Cancel", "More Information", "Create Project", "Copy Project", "Update Warning", "Update Available Samples", "Select Available Sample", "Load Start Choice", "Show Recommended Sample", "Init Spec Page", "Insert Spec Page", "Stop Spec Page", "Set Control Font", "Focus Previous Selection"]
            n126 = event-data() -> ("CtlRef"=w394:refnum<vi>)  [unwired: 1 in, 3 out]
            n127 = property class="Str"(reference=w394, "Text.FontUnder"=TRUE ("Text.Font:Underline")) -> ()  [unwired: 1 in, 2 out]
            n128 = call-poly <vilib>:"Set Cursor.vi"("icon"=u16 6) -> ()  [unwired: 9 in, 2 out]
          }
          event "More Information": Mouse Leave {
            w398 = T4[] [enum."Idle"] items=["Idle", "Initialize", "Parse Config Files", "Update Title", "Update Navigation", "Update Tab", "Load Question", "Load All Samples", "Update Sample Description", "Load Available Samples", "Cancel", "More Information", "Create Project", "Copy Project", "Update Warning", "Update Available Samples", "Select Available Sample", "Load Start Choice", "Show Recommended Sample", "Init Spec Page", "Insert Spec Page", "Stop Spec Page", "Set Control Font", "Focus Previous Selection"]
            n129 = event-data() -> ("CtlRef"=w400:refnum<vi>)  [unwired: 1 in, 3 out]
            n130 = property class="Str"(reference=w400, "Text.FontUnder"=FALSE ("Text.Font:Underline")) -> ()  [unwired: 1 in, 2 out]
            n131 = call-poly <vilib>:"Set Cursor.vi"("icon"=u16 7) -> ()  [unwired: 9 in, 2 out]
          }
          event "More Information": Mouse Up {
            w403 = T4[] [enum."More Information", enum."Idle"] items=["Idle", "Initialize", "Parse Config Files", "Update Title", "Update Navigation", "Update Tab", "Load Question", "Load All Samples", "Update Sample Description", "Load Available Samples", "Cancel", "More Information", "Create Project", "Copy Project", "Update Warning", "Update Available Samples", "Select Available Sample", "Load Start Choice", "Show Recommended Sample", "Init Spec Page", "Insert Spec Page", "Stop Spec Page", "Set Control Font", "Focus Previous Selection"]
            n132 = event-data() -> ()  [unwired: 1 in, 8 out]
          }
          event User Event {
            w412 = T4[] [enum."Update Navigation", enum."Update Warning", enum."Idle"] items=["Idle", "Initialize", "Parse Config Files", "Update Title", "Update Navigation", "Update Tab", "Load Question", "Load All Samples", "Update Sample Description", "Load Available Samples", "Cancel", "More Information", "Create Project", "Copy Project", "Update Warning", "Update Available Samples", "Select Available Sample", "Load Start Choice", "Show Recommended Sample", "Init Spec Page", "Insert Spec Page", "Stop Spec Page", "Set Control Font", "Focus Previous Selection"]
            n133 = event-data() -> ("Errors"=w410:string[])  [unwired: 1 in]
            n134 = Empty Array?(array=w410) -> (empty?=w411:bool)
            n135 = case shown="False" w411 {
              tunnel: w410 -> [w415 _]
              tunnel: [Navigation_Control."Back Enable&Finish Disable" ("Enum") Navigation_Control."Back Enable&Finish" ("Enum")] -> w407
              tunnel: [w416 _] -> w406
              frame False {
                # "If error occurs, disable Finish"
                n136 = call-by-ref "?"("Errors"=w415) -> ("String"=w416:string)  [unwired: 12 in, 2 out]
              }
              frame True {
                # "No errors at this time, so enable the Finish button and empty error text."
              }
            }
            n137 = Bundle By Name(cluster=w409, "Warning"=w406, "Navigation Status"=w407) -> (w408:T5)
          }
          event Key Down? {
            n138 = event-data() -> ("VKey"=w426:T13, "Char"=w425:i16, "PlatMods.Shift"=w433:bool)  [unwired: 1 in]
            n139 = Unbundle By Name(w421) -> ("Selected Sample"=w424:i32, "Available Items"=w422:T3[])
            n140 = Unbundle By Name(w431) -> ("CurPage Ctrl #1"=w430:refnum<vi>, "CurPage Ctrl #n"=w429:refnum<vi>)
            n141 = case shown="\"Start Page\"" w427 {
              tunnel: w425 -> [_ _ _ w476]
              tunnel: w435 -> [_ _ _ w475]
              tunnel: w434 -> [_ _ _ w474]
              tunnel: w426 -> [w441 _ w461 w473]
              tunnel: w433 -> [_ _ _ w472]
              tunnel: w432 -> [_ _ _ w471]
              tunnel: w430 -> [_ _ _ w470]
              tunnel: w429 -> [_ _ _ w469]
              tunnel: [FALSE FALSE FALSE w468] -> w428
              tunnel: w424 -> [w442 w456 w459 w467]
              tunnel: w423 -> [w440 _ _ _]
              tunnel: w422 -> [w439 _ _ _]
              tunnel: [w437 w456 w459 w467] -> w419
              tunnel: [w436 w455 w458 w466] -> w418
              frame "Select Sample" {
                # "up-down arrow to select items"
                n142 = property on="Sample Project" class="Clust (strict)"() -> ("Key Focus"=w443:bool)  [unwired: 2 in, 2 out]
                n143 = Array Size(array=w439) -> (size(s)=w438:i32)
                n144 = case shown="True" w443 {
                  tunnel: w442 -> [w446 w454]
                  tunnel: w441 -> [_ w452]
                  tunnel: w440 -> [_ w451]
                  tunnel: w438 -> [_ w450]
                  tunnel: [w446 w449] -> w437
                  tunnel: [w445 w447] -> w436
                  frame False {
                    w445 = T4[] [enum."Idle"] items=["Idle", "Initialize", "Parse Config Files", "Update Title", "Update Navigation", "Update Tab", "Load Question", "Load All Samples", "Update Sample Description", "Load Available Samples", "Cancel", "More Information", "Create Project", "Copy Project", "Update Warning", "Update Available Samples", "Select Available Sample", "Load Start Choice", "Show Recommended Sample", "Init Spec Page", "Insert Spec Page", "Stop Spec Page", "Set Control Font", "Focus Previous Selection"]
                  }
                  frame True {
                    w447 = T4[] [enum."Select Available Sample", enum."Update Sample Description", enum."Idle"] items=["Idle", "Initialize", "Parse Config Files", "Update Title", "Update Navigation", "Update Tab", "Load Question", "Load All Samples", "Update Sample Description", "Load Available Samples", "Cancel", "More Information", "Create Project", "Copy Project", "Update Warning", "Update Available Samples", "Select Available Sample", "Load Start Choice", "Show Recommended Sample", "Init Spec Page", "Insert Spec Page", "Stop Spec Page", "Set Control Font", "Focus Previous Selection"]
                    n145 = property on="Scrollbar" class="Scroll (strict)"() -> ("Value"=w453:i32)  [unwired: 2 in, 2 out]
                    n146 = call "Sample Up Down.vi"("# Displayed Samples"=w451, "#  Available Samples"=w450, "Selected Sample in"=w454, "VKey"=w452, "Scrollbar Value in"=w453) -> ("Selected Sample out"=w449:i32, "Scrollbar Value out"=w448:i32)  [unwired: 5 in]
                    n147 = property on="Scrollbar" class="Scroll (strict)"("Val(Sgnl)"=w448) -> ()  [unwired: 2 in, 2 out]
                  }
                }
              }
              frame Default {
                w455 = T4[] [enum."Idle"] items=["Idle", "Initialize", "Parse Config Files", "Update Title", "Update Navigation", "Update Tab", "Load Question", "Load All Samples", "Update Sample Description", "Load Available Samples", "Cancel", "More Information", "Create Project", "Copy Project", "Update Warning", "Update Available Samples", "Select Available Sample", "Load Start Choice", "Show Recommended Sample", "Init Spec Page", "Insert Spec Page", "Stop Spec Page", "Set Control Font", "Focus Previous Selection"]
              }
              frame "Start Page" {
                w458 = T4[] [enum."Idle"] items=["Idle", "Initialize", "Parse Config Files", "Update Title", "Update Navigation", "Update Tab", "Load Question", "Load All Samples", "Update Sample Description", "Load Available Samples", "Cancel", "More Information", "Create Project", "Copy Project", "Update Warning", "Update Available Samples", "Select Available Sample", "Load Start Choice", "Show Recommended Sample", "Init Spec Page", "Insert Spec Page", "Stop Spec Page", "Set Control Font", "Focus Previous Selection"]
                n148 = case shown="\"Return\"" w461 {
                  frame "ASCII", Default {
                  }
                  frame "Return" {
                    n149 = property on="Choice 2" class="myRIO Choice Button (strict)"() -> ("Key Focus"=w463:bool)  [unwired: 2 in, 2 out]
                    n150 = property on="Choice 1" class="myRIO Choice Button (strict)"() -> ("Key Focus"=w462:bool)  [unwired: 2 in, 2 out]
                    n151 = case shown="True" w463 {
                      selector: w463 -> [_ w465]
                      frame False {
                      }
                      frame True {
                        n152 = property on="Choice 2" class="myRIO Choice Button (strict)"("Val(Sgnl)"=w465) -> ()  [unwired: 2 in, 2 out]
                      }
                    }
                    n153 = case shown="True" w462 {
                      selector: w462 -> [_ w464]
                      frame False {
                      }
                      frame True {
                        n154 = property on="Choice 1" class="myRIO Choice Button (strict)"("Val(Sgnl)"=w464) -> ()  [unwired: 2 in, 2 out]
                      }
                    }
                  }
                }
              }
              frame "Configure Project" {
                w466 = T4[] [enum."Idle"] items=["Idle", "Initialize", "Parse Config Files", "Update Title", "Update Navigation", "Update Tab", "Load Question", "Load All Samples", "Update Sample Description", "Load Available Samples", "Cancel", "More Information", "Create Project", "Copy Project", "Update Warning", "Update Available Samples", "Select Available Sample", "Load Start Choice", "Show Recommended Sample", "Init Spec Page", "Insert Spec Page", "Stop Spec Page", "Set Control Font", "Focus Previous Selection"]
                # "Tab to select controls"
                n155 = call-by-ref "Call By Reference"("CurPage Ctrl #n"=w469, "Char"=w476, "CurPage Ctrl #1"=w470, "Shift"=w472, "Help"=w471, "Next"=w474, "Back"=w475) -> ("Discard Key Down Event?"=w479:bool)  [unwired: 6 in, 2 out]
                n156 = Not Equal?(x=eventvkey."F1", y=w473) -> (x != y?=w478:bool)
                n157 = And(x=w478, y=w479) -> (x .and. y?=w468:bool)
              }
            }
            n158 = Bundle By Name(cluster=w421, "Selected Sample"=w419) -> (w420:T5)
            n159 = event-data("Discard?"=w428) -> ()  [unwired: 1 in, 1 out]
          }
          event "Choice 1", "Choice 2": Value Change {
            w501 = T4[] [enum."Idle"] items=["Idle", "Initialize", "Parse Config Files", "Update Title", "Update Navigation", "Update Tab", "Load Question", "Load All Samples", "Update Sample Description", "Load Available Samples", "Cancel", "More Information", "Create Project", "Copy Project", "Update Warning", "Update Available Samples", "Select Available Sample", "Load Start Choice", "Show Recommended Sample", "Init Spec Page", "Insert Spec Page", "Stop Spec Page", "Set Control Font", "Focus Previous Selection"]
            n160 = event-data() -> ("CtlRef"=w498:refnum<vi>)  [unwired: 1 in, 2 out]
            n161 = control-ref of="Choice 1"() -> (w499:refnum<vi>)
            n162 = Unbundle By Name(w503) -> ("Selected Choices"=w500:T7[], "Current Choice Index"=w495:i32, "Question List"=w489:T11[])
            n163 = Generate User Event(user event=w505, event data cluster=TRUE ("event data")) -> ()  [unwired: 2 in, 2 out]
            n164 = Unbundle By Name(w494) -> ("Selected Question"=w488:i32)
            n165 = Equal?(x=w499, y=w498) -> (x = y?=w490:bool)
            n166 = Index Array(array=w500, index #1=w495) -> (element #1=w497:T7, element #2=w496:T7)  [unwired: 1 in]
            n167 = Index Array(array=w489, index=w488) -> (element=w487:T11)
            n168 = case shown="True" w490 {
              tunnel: w497 -> [w516 w529]
              tunnel: w496 -> [w515 w527]
              tunnel: [w514 w528] -> w481
              tunnel: w495 -> [w513 w536]
              tunnel: w500 -> [w512 w537]
              tunnel: [w511 w535] -> w491
              tunnel: w487 -> [w510 w534]
              tunnel: [Answers."Choice 1" ("Answers") Answers."Choice 2" ("Answers")] -> w486
              tunnel: [w508 w532] -> w485
              tunnel: [w507 w531] -> w482
              tunnel: [w506 w530] -> w484
              frame True {
                # "Select Choice1"
                n169 = case shown="\"Choice 2\"" w516 {
                  tunnel: w515 -> [w520 _]
                  tunnel: [w518 TRUE] -> w514
                  tunnel: w513 -> [_ w523]
                  tunnel: w512 -> [w517 w526]
                  tunnel: [w517 w522] -> w511
                  frame "Choice 1", Default {
                    # "used to select Choice1--> come to next selection and update the list \nelse load default status"
                    n170 = Equal?(x=Answers."Choice 1" ("Answers"), y=w520) -> (x = y?=w518:bool)
                  }
                  frame "Choice 2" {
                    # "Used to select Choice2-->\nclear the list"
                    n171 = Replace Array Subset(array=w526, new element=Answers."Choice 1" ("element"), index=w523) -> (w524:T7[])
                    n172 = call "Clear Follow Record.vi"("Current Choice Index"=w523, "Selected Choices"=w524) -> ("Selected Choices Out"=w522:T7[])  [unwired: 9 in]
                  }
                }
                n173 = Unbundle By Name(w510) -> ("Choice 1.ReachSample"=w508:bool, "Choice 1.NextQuestion"=w507:i32, "Choice 1.Sample"=w506:string)
              }
              frame False {
                # "Select Choice2"
                n174 = case shown="\"Choice 2\"" w529 {
                  tunnel: w537 -> [w541 w545]
                  tunnel: w536 -> [w540 _]
                  tunnel: [w539 w545] -> w535
                  tunnel: [TRUE w544] -> w528
                  tunnel: w527 -> [_ w546]
                  frame "Choice 1", Default {
                    # "Used to select Choice1, update and clear list"
                    n175 = Replace Array Subset(array=w541, new element=Answers."Choice 2" ("element"), index=w540) -> (w542:T7[])
                    n176 = call "Clear Follow Record.vi"("Current Choice Index"=w540, "Selected Choices"=w542) -> ("Selected Choices Out"=w539:T7[])  [unwired: 9 in]
                  }
                  frame "Choice 2" {
                    # "Used to select Choice2, load next question status"
                    n177 = Equal?(x=Answers."Choice 1" ("Answers"), y=w546) -> (x = y?=w544:bool)
                  }
                }
                n178 = Unbundle By Name(w534) -> ("Choice 2.ReachSample"=w532:bool, "Choice 2.NextQuestion"=w531:i32, "Choice 2.Sample"=w530:string)
              }
            }
            n179 = Increment(x=w495) -> (x+1=w492:i32)
            n180 = Not(x=w481) -> (.not. x?=w480:bool)
            n181 = property on="Choice 1" class="myRIO Choice Button (strict)"("Value"=w481) -> ()  [unwired: 2 in, 2 out]
            n182 = property on="Choice 2" class="myRIO Choice Button (strict)"("Value"=w480) -> ()  [unwired: 2 in, 2 out]
            n183 = Not(x=w485) -> (.not. x?=w483:bool)
            n184 = Bundle By Name(cluster=w494, "Answers"=w486, "Result"=w484) -> (w493:T5)
            n185 = Bundle By Name(cluster=w503, "Have Next Page"=w483, "Next Page\n Index"=w482, "Selected Choices"=w491, "Current Choice Index"=w492) -> (w502:T8)
          }
        }
      }
      frame "Initialize" {
        w548 = T7[] [enum."Choice 1", enum."Choice 1", enum."Choice 1", enum."Choice 1", enum."Choice 1", enum."Choice 1", enum."Choice 1", enum."Choice 1"] items=["Choice 1", "Choice 2"] ("Selected Choices")
        w564 = T4[] [enum."Parse Config Files", enum."Update Title", enum."Update Navigation", enum."Update Tab", enum."Update Warning", enum."Set Control Font", enum."Update Available Samples", enum."Load Start Choice", enum."Idle"] items=["Idle", "Initialize", "Parse Config Files", "Update Title", "Update Navigation", "Update Tab", "Load Question", "Load All Samples", "Update Sample Description", "Load Available Samples", "Cancel", "More Information", "Create Project", "Copy Project", "Update Warning", "Update Available Samples", "Select Available Sample", "Load Start Choice", "Show Recommended Sample", "Init Spec Page", "Insert Spec Page", "Stop Spec Page", "Set Control Font", "Focus Previous Selection"]
        # "Preallocate the Selected Choice"
        # "Initialize Project"
        n186 = Bundle By Name(cluster=w553, "Current Choice Index"=0 ("Selection Index"), "Selected Choices"=w548) -> (w550:T8)
        n187 = Bundle By Name(cluster=w559, "Show Guidance"=TRUE, "Warning"="", "Title Index"=0, "Navigation Status"=Navigation_Control."Back Disable&Next Disable", "Tab Control"=Tab_Control."Start Page", "Answers"=Answers."Choice 1") -> (w560:T5)
      }
      frame "Set Control Font" {
        w571 = T4[] [] items=["Idle", "Initialize", "Parse Config Files", "Update Title", "Update Navigation", "Update Tab", "Load Question", "Load All Samples", "Update Sample Description", "Load Available Samples", "Cancel", "More Information", "Create Project", "Copy Project", "Update Warning", "Update Available Samples", "Select Available Sample", "Load Start Choice", "Show Recommended Sample", "Init Spec Page", "Insert Spec Page", "Stop Spec Page", "Set Control Font", "Focus Previous Selection"]
        n188 = property on="Sample Project" class="Clust (strict)"() -> ("Controls[]"=w570:refnum<vi>[])  [unwired: 2 in, 2 out]
        n189 = for {
          tunnel: w570 -> [w602] mode=indexing
          w586 = u32 0
          w580 = u32 15 ("Text.Font:Size")
          n190 = control-ref of="List Item"() -> (w601:refnum<vi>)
          n191 = To More Specific Class(target class=w601, reference=w602) -> (specific class reference=w600:refnum<vi>, error out=w599:errorcluster)  [unwired: 1 in]
          n192 = property class="Clust (strict)"(reference=w600, error in=w599) -> ("Controls[]"=w598:refnum<vi>[])  [unwired: 2 out]
          n193 = control-ref of="Name"() -> (w597:refnum<vi>)
          n194 = control-ref of="More Info"() -> (w588:refnum<vi>)
          n195 = control-ref of="Description"() -> (w590:refnum<vi>)
          n196 = Index Array(array=w598) -> (element #1=w596:refnum<vi>, element #2=w591:refnum<vi>, element #3=w589:refnum<vi>)  [unwired: 3 in]
          n197 = To More Specific Class(target class=w597, reference=w596) -> (specific class reference=w595:refnum<vi>)  [unwired: 1 in, 1 out]
          n198 = To More Specific Class(target class=w590, reference=w591) -> (specific class reference=w592:refnum<vi>)  [unwired: 1 in, 1 out]
          n199 = To More Specific Class(target class=w588, reference=w589) -> (specific class reference=w584:refnum<vi>)  [unwired: 1 in, 1 out]
          n200 = call <vilib>:"Hilite Color.vi"("Percentage(30)"=50.0, "Color In"=w586) -> ("Hilite"=w582:u32)  [unwired: 1 out]
          n201 = call <vilib>:"Hilite Color.vi"("Percentage(30)"=30.0, "Color In"=w586) -> ("Hilite"=w585:u32)  [unwired: 1 out]
          n202 = property class="Str"(reference=w595, "Text.FontName"="Applicatoin Font" ("Text.Font:Name"), "Text.FontSize"=w580, "Text.TextColor"=w586, "Text.FontBold"=TRUE ("Text.Font:Bold")) -> ()  [unwired: 1 in, 2 out]
          n203 = property class="Str"(reference=w584, "Text.TextColor"=w585, "Text.FontBold"=TRUE ("Text.Font:Bold"), "Text.FontSize"=w580) -> ()  [unwired: 1 in, 2 out]
          n204 = property class="Str"(reference=w592, "Text.TextColor"=w582, "Text.FontBold"=FALSE ("Text.Font:Bold"), "Text.FontSize"=w580) -> ()  [unwired: 1 in, 2 out]
        }
        n205 = call <vilib>:"Hilite Color.vi"("Percentage(30)"=30.0, "Color In"=u32 0) -> ("Hilite"=w566:u32)  [unwired: 1 out]
        n206 = property on="More Information" class="Str"("Text.FontBold"=TRUE ("Text.Font:Bold"), "Text.TextColor"=w566) -> ()  [unwired: 2 in, 2 out]
      }
      frame "Parse Config Files" {
        w604 = T4[] [] items=["Idle", "Initialize", "Parse Config Files", "Update Title", "Update Navigation", "Update Tab", "Load Question", "Load All Samples", "Update Sample Description", "Load Available Samples", "Cancel", "More Information", "Create Project", "Copy Project", "Update Warning", "Update Available Samples", "Select Available Sample", "Load Start Choice", "Show Recommended Sample", "Init Spec Page", "Insert Spec Page", "Stop Spec Page", "Set Control Font", "Focus Previous Selection"]
        n207 = in-place {
          in-place-border: w609 -> [w622]
          in-place-border: [w619] -> w608
          in-place-border: w603 -> [w615]
          # "Load configure files"
          n208 = in-place-cluster #2(w612) -> ("Item List"=w630:T9, "Question List"=w625:T11[])
          n209 = Format Into String(format string="Config File\\\\%s\\\\Questions.xml", w615) -> (resulting string=w616:string)  [unwired: 2 in, 1 out]
          n210 = Format Into String(format string="Config File\\\\%s\\\\Item List Info.xml", w615) -> (resulting string=w617:string)  [unwired: 2 in, 1 out]
          n211 = Current VI's Path() -> (path=w634:path)
          n212 = Strip Path(path=w634) -> (stripped path=w623:path)  [unwired: 1 out]
          n213 = Build Path(base path=w623, name or relative path=w616) -> (appended path=w626:path)
          n214 = Build Path(base path=w623, name or relative path=w617) -> (appended path=w633:path)
          n215 = call-poly <vilib>:"Read From XML File.vi"("error in (no error)"=w622, "XML File Path"=w626) -> ("error out"=w628:errorcluster, "XML Elements"=w627:string)  [unwired: 7 in, 1 out]
          n216 = call-poly <vilib>:"Read From XML File.vi"("error in (no error)"=w622, "XML File Path"=w633) -> ("error out"=w631:errorcluster, "XML Elements"=w632:string)  [unwired: 7 in, 1 out]
          n217 = Unflatten From XML(xml string=w627, type=w625, error in (no error)=w628) -> (value=w624:T11[], error out=w620:errorcluster)
          n218 = Unflatten From XML(xml string=w632, type=w630, error in (no error)=w631) -> (value=w629:T9, error out=w621:errorcluster)
          n219 = Merge Errors(w621, w620) -> (w619:errorcluster)
          n220 = in-place-cluster #2("Item List"=w629, "Question List"=w624) -> (w611:T8)
        }
      }
      frame "Update Title" {
        w635 = T4[] [] items=["Idle", "Initialize", "Parse Config Files", "Update Title", "Update Navigation", "Update Tab", "Load Question", "Load All Samples", "Update Sample Description", "Load Available Samples", "Cancel", "More Information", "Create Project", "Copy Project", "Update Warning", "Update Available Samples", "Select Available Sample", "Load Start Choice", "Show Recommended Sample", "Init Spec Page", "Insert Spec Page", "Stop Spec Page", "Set Control Font", "Focus Previous Selection"]
        n221 = Unbundle By Name(w641) -> ("Title Index"=w639:i32)
        n222 = Index Array(array=string[] ["Answer questions to choose a sample project:", "", "Choose a sample:", "Configure the new project:"] ("Title Name"), index=w639) -> ()  [unwired: 1 out]
      }
      frame "Update Navigation" {
        w645 = T4[] [] items=["Idle", "Initialize", "Parse Config Files", "Update Title", "Update Navigation", "Update Tab", "Load Question", "Load All Samples", "Update Sample Description", "Load Available Samples", "Cancel", "More Information", "Create Project", "Copy Project", "Update Warning", "Update Available Samples", "Select Available Sample", "Load Start Choice", "Show Recommended Sample", "Init Spec Page", "Insert Spec Page", "Stop Spec Page", "Set Control Font", "Focus Previous Selection"]
        n223 = Unbundle By Name(w651) -> ("Navigation Status"=w652:T6)
        n224 = call "Set Navigation.vi"("Enum"=w652, "Back"=w649, "Next"=w648) -> ()  [unwired: 9 in]
      }
      frame "Update Tab" {
        w656 = T4[] [] items=["Idle", "Initialize", "Parse Config Files", "Update Title", "Update Navigation", "Update Tab", "Load Question", "Load All Samples", "Update Sample Description", "Load Available Samples", "Cancel", "More Information", "Create Project", "Copy Project", "Update Warning", "Update Available Samples", "Select Available Sample", "Load Start Choice", "Show Recommended Sample", "Init Spec Page", "Insert Spec Page", "Stop Spec Page", "Set Control Font", "Focus Previous Selection"]
        n225 = Unbundle By Name(w660) -> ("Tab Control"=w661:T1)
        n226 = property on="Tab Control" class="TabCtl (strict)"("Value"=w661) -> ()  [unwired: 2 in, 2 out]
      }
      frame "Load Question" {
        w675 = T4[] [] items=["Idle", "Initialize", "Parse Config Files", "Update Title", "Update Navigation", "Update Tab", "Load Question", "Load All Samples", "Update Sample Description", "Load Available Samples", "Cancel", "More Information", "Create Project", "Copy Project", "Update Warning", "Update Available Samples", "Select Available Sample", "Load Start Choice", "Show Recommended Sample", "Init Spec Page", "Insert Spec Page", "Stop Spec Page", "Set Control Font", "Focus Previous Selection"]
        # "Update question"
        n227 = Unbundle By Name(w681) -> ("Selected Question"=w692:i32)
        n228 = Unbundle By Name(w688) -> ("Question List"=w693:T11[])
        n229 = Index Array(array=w693, index=w692) -> (element=w690:T11)
        n230 = Unbundle By Name(w690) -> ("Choice 1"=w686:T12, "Text"=→"Question":string, "Choice 1.Text"=w673:string, "Choice 2.Text"=w671:string)
        n231 = Pick Line(multi-line string=w673, line index=0) -> (output string=w674:string)  [unwired: 1 in]
        n232 = Pick Line(multi-line string=w673, line index=1) -> (output string=w672:string)  [unwired: 1 in]
        n233 = Pick Line(multi-line string=w671, line index=0) -> (output string=w666:string)  [unwired: 1 in]
        n234 = Pick Line(multi-line string=w671, line index=1) -> (output string=w665:string)  [unwired: 1 in]
        n235 = Unbundle By Name(w686) -> ("Sample"=w682:string, "ReachSample"=w683:bool, "NextQuestion"=w685:i32)
        n236 = property on="Choice 2" class="myRIO Choice Button (strict)"("Title"=w666, "Explanation"=w665) -> ()  [unwired: 2 in, 2 out]
        n237 = property on="Choice 1" class="myRIO Choice Button (strict)"("Title"=w674, "Explanation"=w672) -> ()  [unwired: 2 in, 2 out]
        n238 = Not(x=w683) -> (.not. x?=w684:bool)
        n239 = Bundle By Name(cluster=w688, "Have Next Page"=w684, "Next Page\n Index"=w685) -> (w687:T8)
        n240 = Bundle By Name(cluster=w681, "Answers"=Answers."Choice 1", "Result"=w682) -> (w680:T5)
      }
      frame "Focus Previous Selection" {
        w696 = T4[] [] items=["Idle", "Initialize", "Parse Config Files", "Update Title", "Update Navigation", "Update Tab", "Load Question", "Load All Samples", "Update Sample Description", "Load Available Samples", "Cancel", "More Information", "Create Project", "Copy Project", "Update Warning", "Update Available Samples", "Select Available Sample", "Load Start Choice", "Show Recommended Sample", "Init Spec Page", "Insert Spec Page", "Stop Spec Page", "Set Control Font", "Focus Previous Selection"]
        n241 = Unbundle By Name(w700) -> ("Previous Selection"=w699:T7)
        n242 = Equal?(x=w699, y=Answers."Choice 1") -> (x = y?=w698:bool)
        n243 = Not(x=w698) -> (.not. x?=w697:bool)
        n244 = property on="Choice 1" class="myRIO Choice Button (strict)"("Value"=w698) -> ()  [unwired: 2 in, 2 out]
        n245 = property on="Choice 2" class="myRIO Choice Button (strict)"("Value"=w697) -> ()  [unwired: 2 in, 2 out]
      }
      frame "Load All Samples" {
        w708 = T4[] [] items=["Idle", "Initialize", "Parse Config Files", "Update Title", "Update Navigation", "Update Tab", "Load Question", "Load All Samples", "Update Sample Description", "Load Available Samples", "Cancel", "More Information", "Create Project", "Copy Project", "Update Warning", "Update Available Samples", "Select Available Sample", "Load Start Choice", "Show Recommended Sample", "Init Spec Page", "Insert Spec Page", "Stop Spec Page", "Set Control Font", "Focus Previous Selection"]
        w707 = 0 ("Selected Sample")
        n246 = control-ref of="Category:"() -> (w714:refnum<vi>)
        n247 = Unbundle By Name(w716) -> ("Item List"=w715:T9)
        n248 = call "Load Sample Catagory.vi"("error in (no error)"=w713, "Item List"=w715, "TreeControl in"=w714) -> ("error out"=w712:errorcluster)  [unwired: 8 in]
        n249 = Bundle By Name(cluster=w719, "Scrollbar Value"=w707, "Selected Sample"=w707, "Sample Filter"="") -> (w718:T5)
      }
      frame "Update Sample Description" {
        w722 = T4[] [] items=["Idle", "Initialize", "Parse Config Files", "Update Title", "Update Navigation", "Update Tab", "Load Question", "Load All Samples", "Update Sample Description", "Load Available Samples", "Cancel", "More Information", "Create Project", "Copy Project", "Update Warning", "Update Available Samples", "Select Available Sample", "Load Start Choice", "Show Recommended Sample", "Init Spec Page", "Insert Spec Page", "Stop Spec Page", "Set Control Font", "Focus Previous Selection"]
        n250 = Unbundle By Name(w733) -> ("Sample Item Names"=w729:string[], "Item List"=w732:T9)
        n251 = Unbundle By Name(w726) -> ("Selected Sample"=w730:i32)
        n252 = Index Array(array=w729, index=w730) -> (element=w728:string)
        n253 = call "Get Template Page.vi"("Target Name"=w721, "error in (no error)"=w727, "Item List"=w732, "Item Name"=w728) -> ("error out"=w734:errorcluster, "picture"=→"Sample Pic":picture)  [unwired: 4 in, 2 out]
      }
      frame "Load Available Samples" {
        w744 = T4[] [enum."Select Available Sample"] items=["Idle", "Initialize", "Parse Config Files", "Update Title", "Update Navigation", "Update Tab", "Load Question", "Load All Samples", "Update Sample Description", "Load Available Samples", "Cancel", "More Information", "Create Project", "Copy Project", "Update Warning", "Update Available Samples", "Select Available Sample", "Load Start Choice", "Show Recommended Sample", "Init Spec Page", "Insert Spec Page", "Stop Spec Page", "Set Control Font", "Focus Previous Selection"]
        n254 = Unbundle By Name(w753) -> ("Sample Filter"=w742:string)
        n255 = control-ref of="Scrollbar"() -> (w757:refnum<vi>)
        n256 = Unbundle By Name(w760) -> ("Item List"=w758:T9)
        n257 = case shown="\"\"" w742 {
          selector: w742 -> [_ w767]
          tunnel: w761 -> [w765 w771]
          tunnel: [w764 w770] -> w738
          tunnel: w758 -> [w766 w769]
          tunnel: [w763 w768] -> w756
          frame "" {
            n258 = call "Get All Leaves by Itemlist.vi"("error in"=w765, "Item List"=w766) -> ("error IO"=w764:errorcluster, "Children Tags"=w763:string[])  [unwired: 8 in]
          }
          frame Default {
            n259 = call "Get Child Leaves by Itemlist.vi"("error in"=w771, "Item List"=w769, "Parent Tag"=w767) -> ("error IO"=w770:errorcluster, "Children Tags"=w768:string[])  [unwired: 7 in]
          }
        }
        n260 = Array Size(array=w756) -> (size(s)=w755:i32)
        n261 = call "Set Artificial Scrollbar.vi"("error in (no error)"=w738, "# Displayed Items"=w737, "Array Size"=w755, "Scrollbar in"=w757) -> ("error IO"=w754:errorcluster)  [unwired: 7 in]
        n262 = for {
          tunnel: w756 -> [w786] mode=indexing
          tunnel: w758 -> [w788]
          shift-right: [w784] -> w751
          shift-left: w754 -> [w787]
          tunnel: [w783] -> w746 mode=indexing
          tunnel: w736 -> [w781]
          n263 = call "Get Template Page.vi"("Target Name"=w781, "error in (no error)"=w787, "Item List"=w788, "Item Name"=w786) -> ("error out"=w784:errorcluster, "Description"=w785:string)  [unwired: 4 in, 2 out]
          n264 = Bundle By Name(cluster=T3 {"Name"="", "Description"="", "More Info"="More Information"} ("List Item"), "Name"=w786, "Description"=w785) -> (w783:T3)
        }
        n265 = Array Size(array=w746) -> (size(s)=w749:i32)
        n266 = Bundle By Name(cluster=w753, "Available Items"=w746, "Selected Sample"=0) -> (w752:T5)
        n267 = Subtract(x=w737, y=w749) -> (x-y=w747:i32)
        n268 = Greater?(x=w747, y=0) -> (0:w750:bool)
        n269 = case shown="True" w750 {
          tunnel: w746 -> [w774 w777]
          tunnel: [w773 w778] -> w745
          tunnel: w747 -> [_ w779]
          tunnel: w737 -> [w772 _]
          frame False {
            # "only display 5 Item"
            n270 = for {
              N: w772 -> [_]
              tunnel: w774 -> [w775] mode=indexing
              tunnel: [w775] -> w773 mode=indexing
            }
          }
          frame True {
            # "less than four Items, fill it."
            n271 = for {
              N: w779 -> [_]
              tunnel: [T3 {"Name"="", "Description"="", "More Info"=""} ("List Item")] -> w776 mode=indexing
            }
            n272 = Insert Into Array(array=w777, new element=w776) -> (w778:T3[])  [unwired: 1 in]
          }
        }
        n273 = Bundle By Name(cluster=w760, "Displayed Available Sample"=w745, "Sample Item Names"=w756) -> (w759:T8)
      }
      frame "Cancel" {
        w789 = T4[] [] items=["Idle", "Initialize", "Parse Config Files", "Update Title", "Update Navigation", "Update Tab", "Load Question", "Load All Samples", "Update Sample Description", "Load Available Samples", "Cancel", "More Information", "Create Project", "Copy Project", "Update Warning", "Update Available Samples", "Select Available Sample", "Load Start Choice", "Show Recommended Sample", "Init Spec Page", "Insert Spec Page", "Stop Spec Page", "Set Control Font", "Focus Previous Selection"]
        n274 = Unbundle By Name(w795) -> ("Spec Page Reference"=w790:refnum<vi>)
        n275 = Not A Number/Path/Refnum?(number/path/refnum=w790) -> (NaN/Path/Refnum?=w791:bool)
        n276 = case shown="False" w791 {
          tunnel: w794 -> [w809 w810]
          tunnel: [w808 w810] -> w793
          tunnel: w790 -> [w805 _]
          frame False {
            n277 = invoke class="VI" method="Abort VI"(reference=w805, error in=w809) -> (reference out=w807:refnum<vi>, error out=w806:errorcluster)  [unwired: 1 in, 1 out]
            n278 = Close Reference(reference=w807, error in (no error)=w806) -> (error out=w808:errorcluster)
          }
          frame True {
          }
        }
        n279 = call-dynamic "Fire Quit Event.vi"("error in (no error)"=w793, "Force Quit?"=TRUE, "BaseSpecPage in"=w797) -> ("error out"=w800:errorcluster, "BaseSpecPage out"=w799:refnum<class "BaseSpecPage.lvclass">)  [unwired: 6 in, 1 out]
        n280 = call-dynamic "Finalize.vi"("error in (no error)"=w800, "BaseSpecPage in"=w799) -> ("error out"=w792:errorcluster)  [unwired: 7 in, 2 out]
      }
      frame "More Information" {
        w833 = T4[] [] items=["Idle", "Initialize", "Parse Config Files", "Update Title", "Update Navigation", "Update Tab", "Load Question", "Load All Samples", "Update Sample Description", "Load Available Samples", "Cancel", "More Information", "Create Project", "Copy Project", "Update Warning", "Update Available Samples", "Select Available Sample", "Load Start Choice", "Show Recommended Sample", "Init Spec Page", "Insert Spec Page", "Stop Spec Page", "Set Control Font", "Focus Previous Selection"]
        n281 = Unbundle By Name(w827) -> ("Sample Item Names"=w826:string[], "Item List"=w825:T9)
        n282 = Unbundle By Name(w828) -> ("Result"=w832:string, "Show Guidance"=w831:bool, "Selected Sample"=w830:i32)
        n283 = case shown="False" w831 {
          tunnel: [w845 w846] -> w829
          tunnel: w826 -> [w844 _]
          tunnel: w832 -> [_ w846]
          tunnel: w830 -> [w843 _]
          frame False {
            n284 = Index Array(array=w844, index=w843) -> (element=w845:string)
          }
          frame True {
          }
        }
        n285 = call "Find Item By Tag.vi"("Tag"=w829, "Item List"=w825) -> ("Item Info"=w824:T10)  [unwired: 9 in]
        n286 = Current VI's Path() -> (path=w817:path)
        n287 = Unbundle By Name(w824) -> ("Sample Folder Name"=w822:string, "Documentation Name"=w819:string)
        n288 = for {
          N: 3 -> [_]
          shift-right: [w841] -> w815
          shift-left: w817 -> [w842]
          n289 = Strip Path(path=w842) -> (stripped path=w841:path)  [unwired: 1 out]
        }
        n290 = Build Path(base path=w815, name or relative path=w822) -> (appended path=w821:path)
        n291 = Build Path(base path=w821, name or relative path="documentation") -> (appended path=w818:path)
        n292 = Build Path(base path=w818, name or relative path=w819) -> (appended path=w813:path)
        n293 = Not A Number/Path/Refnum?(number/path/refnum=w813) -> (NaN/Path/Refnum?=w814:bool)
        n294 = case shown="True" w814 {
          tunnel: w813 -> [w839 _]
          tunnel: w812 -> [w838 w840]
          tunnel: [w837 w840] -> w811
          frame False {
            n295 = call-poly <vilib>:"Open URL in Default Browser.vi"("error in (no error)"=w838, "path"=w839) -> ("error out"=w837:errorcluster)  [unwired: 4 in, 1 out]
          }
          frame True {
          }
        }
      }
      frame "Create Project" {
        w847 = T4[] [enum."Cancel"] items=["Idle", "Initialize", "Parse Config Files", "Update Title", "Update Navigation", "Update Tab", "Load Question", "Load All Samples", "Update Sample Description", "Load Available Samples", "Cancel", "More Information", "Create Project", "Copy Project", "Update Warning", "Update Available Samples", "Select Available Sample", "Load Start Choice", "Show Recommended Sample", "Init Spec Page", "Insert Spec Page", "Stop Spec Page", "Set Control Font", "Focus Previous Selection"]
        # "Just in case the custom scripting did not close the progress bar, make sure it gets closed"
        # "Tranform path to current root"
        n296 = property class="MetaDataObj.lvclass"(reference=w864) -> (reference out=w863:refnum<class "MetaDataObj.lvclass">, "Custom VI Path"=w854:path)  [unwired: 1 in, 1 out]
        n297 = Unbundle By Name(w862) -> ("User Project"=w851:refnum<vi>)
        n298 = Open VI Reference(type specifier VI Refnum (for type only)=refnum<vi> refnum, vi path=w854, error in (no error)=w850) -> (vi reference=w861:refnum<vi>, error out=w859:errorcluster)  [unwired: 3 in]
        n299 = call-by-ref "?"(reference=w861, error in=w859, "DNL_MetaDataObj"=w863, "Project"=w851) -> (reference out=w858:refnum<vi>, error out=w857:errorcluster)  [unwired: 10 in]
        n300 = Close Reference(reference=w858, error in (no error)=w857) -> (error out=w856:errorcluster)
        n301 = call <vilib>:"Clear Errors.vi"("error in (no error)"=w856) -> ("error out"=w855:errorcluster)  [unwired: 5 in, 1 out]
        n302 = call <resource>:"Close Create Project Progress Bar.vi"("error in (no error)"=w855, "Project"=w851) -> ("error out"=w852:errorcluster, "dup Project"=w853:refnum<vi>)  [unwired: 8 in]
        n303 = Close Reference(reference=w853, error in (no error)=w852) -> (error out=w849:errorcluster)
      }
      frame "Copy Project" {
        n304 = property class="MetaDataObj.lvclass"(reference=w870, error in=w869) -> (reference out=w876:refnum<class "MetaDataObj.lvclass">, error out=w885:errorcluster, "Project Path"=w886:path, "Project Root"=w882:path, "File Prefix"=w881:string, "Project Name"=w880:string, "Overlay Icon"=w879:refnum<class "Icon.lvclass">)
        n305 = Build Array(w882) -> (w887:path[])
        n306 = call-by-ref "?"(error in=w885, "value"=w887, "key"=w871) -> (error out=w884:errorcluster)  [unwired: 6 in, 2 out]
        n307 = call-by-ref "?"(error in=w884, "File Path In"=w886) -> (error out=w883:errorcluster, "Valid File Path?"=w877:bool, "File Path Out"=w878:path)  [unwired: 10 in, 1 out]
        n308 = case shown="True" w877 {
          tunnel: w881 -> [_ w906]
          tunnel: w880 -> [_ w904]
          tunnel: w879 -> [_ _]
          tunnel: w882 -> [_ w905]
          tunnel: w878 -> [_ w903]
          tunnel: w876 -> [_ w902]
          tunnel: w883 -> [w893 w900]
          tunnel: w875 -> [w894 w899]
          tunnel: [w894 w898] -> w874
          tunnel: [w891 w897] -> w873
          tunnel: [w893 w895] -> w872
          frame False {
            w891 = T4[] [enum."Cancel"] items=["Idle", "Initialize", "Parse Config Files", "Update Title", "Update Navigation", "Update Tab", "Load Question", "Load All Samples", "Update Sample Description", "Load Available Samples", "Cancel", "More Information", "Create Project", "Copy Project", "Update Warning", "Update Available Samples", "Select Available Sample", "Load Start Choice", "Show Recommended Sample", "Init Spec Page", "Insert Spec Page", "Stop Spec Page", "Set Control Font", "Focus Previous Selection"]
            n309 = One Button Dialog(message="LabVIEW can't find the source files for this project.") -> ()  [unwired: 1 in, 1 out]
          }
          frame True {
            w897 = T4[] [enum."Create Project"] items=["Idle", "Initialize", "Parse Config Files", "Update Title", "Update Navigation", "Update Tab", "Load Question", "Load All Samples", "Update Sample Description", "Load Available Samples", "Cancel", "More Information", "Create Project", "Copy Project", "Update Warning", "Update Available Samples", "Select Available Sample", "Load Start Choice", "Show Recommended Sample", "Init Spec Page", "Insert Spec Page", "Stop Spec Page", "Set Control Font", "Focus Previous Selection"]
            # "Unwire to avoid overlay icon"
            # "Set a busy cursor... this is the point of no return"
            n310 = call-by-ref "?"(error in=w900) -> ("error out"=w901:errorcluster)  [unwired: 11 in, 3 out]
            n311 = call-by-ref "?"("Target Project Name"=w904, "MetaDataObj"=w902, "error in (no error)"=w901, "Target File Prefix"=w906, "Target Path"=w905, "Source Project Path"=w903) -> (error out=w895:errorcluster, "Project"=w896:refnum<vi>)  [unwired: 6 in, 2 out]
            n312 = Bundle By Name(cluster=w899, "User Project"=w896) -> (w898:T8)
          }
        }
      }
      frame "Update Warning" {
        w907 = T4[] [] items=["Idle", "Initialize", "Parse Config Files", "Update Title", "Update Navigation", "Update Tab", "Load Question", "Load All Samples", "Update Sample Description", "Load Available Samples", "Cancel", "More Information", "Create Project", "Copy Project", "Update Warning", "Update Available Samples", "Select Available Sample", "Load Start Choice", "Show Recommended Sample", "Init Spec Page", "Insert Spec Page", "Stop Spec Page", "Set Control Font", "Focus Previous Selection"]
        n313 = Unbundle By Name(w912) -> ("Warning"=→"Error Messages":string)
      }
      frame "Update Available Samples" {
        w916 = 15
        w941 = T4[] [] items=["Idle", "Initialize", "Parse Config Files", "Update Title", "Update Navigation", "Update Tab", "Load Question", "Load All Samples", "Update Sample Description", "Load Available Samples", "Cancel", "More Information", "Create Project", "Copy Project", "Update Warning", "Update Available Samples", "Select Available Sample", "Load Start Choice", "Show Recommended Sample", "Init Spec Page", "Insert Spec Page", "Stop Spec Page", "Set Control Font", "Focus Previous Selection"]
        n314 = Unbundle By Name(w952) -> ("Displayed Available Sample"=w939:T3[])
        n315 = property on="Description" class="Str"() -> ("Width"=w940:u32)  [unwired: 2 in, 2 out]
        n316 = for {
          tunnel: w939 -> [w959] mode=indexing
          tunnel: w940 -> [w961]
          tunnel: [w958] -> w938 mode=indexing
          tunnel: [w956] -> w937 mode=indexing
          n317 = Unbundle By Name(w959) -> ("More Info"=w957:string, "Description"=w962:string)
          n318 = call "Fit Description.vi"("Word Wrap Bound"=w961, "Description"=w962, "Project Information"=w957) -> ("Description out"=w960:string, "Tail Pos"=w956:u32)  [unwired: 5 in, 2 out]
          n319 = Bundle By Name(cluster=w959, "Description"=w960) -> (w958:T3)
        }
        n320 = Index Array(array=w937) -> (element #1=w917:u32, element #2=w930:u32, element #3=w926:u32, element #4=w919:u32, element #5=w918:u32)  [unwired: 5 in]
        n321 = Index Array(array=w938) -> (element #1=w947:T3, element #2=w946:T3, element #3=w945:T3, element #4=w944:T3, element #5=w943:T3)  [unwired: 5 in]
        n322 = property on="Description" class="Str"() -> ("Position"=w936:T16)  [unwired: 2 in, 2 out]
        n323 = property on="Description" class="Str"() -> ("Position"=w933:T16)  [unwired: 2 in, 2 out]
        n324 = property on="Description" class="Str"() -> ("Position"=w928:T16)  [unwired: 2 in, 2 out]
        n325 = property on="Description" class="Str"() -> ("Position"=w924:T16)  [unwired: 2 in, 2 out]
        n326 = property on="Description" class="Str"() -> ("Position"=w921:T16)  [unwired: 2 in, 2 out]
        n327 = Bundle By Name(cluster=T2 {"List Item"={"Name"="", "Description"="", "More Info"=""}, "List Item 2"={"Name"="", "Description"="", "More Info"=""}, "List Item 3"={"Name"="", "Description"="", "More Info"=""}, "List Item 4"={"Name"="", "Description"="", "More Info"=""}, "List Item 5"={"Name"="", "Description"="", "More Info"=""}} ("Sample Project"), "List Item"=w947, "List Item 2"=w946, "List Item 3"=w945, "List Item 4"=w944, "List Item 5"=w943) -> (w942:T2)
        n328 = Bundle By Name(cluster=w933, "Top"=w916, "Left"=w930) -> (w932:T16)
        n329 = Bundle By Name(cluster=w936, "Top"=w916, "Left"=w917) -> (w935:T16)
        n330 = Bundle By Name(cluster=w928, "Top"=w916, "Left"=w926) -> (w929:T16)
        n331 = Bundle By Name(cluster=w924, "Top"=w916, "Left"=w919) -> (w925:T16)
        n332 = Bundle By Name(cluster=w921, "Top"=w916, "Left"=w918) -> (w922:T16)
        n333 = property on="Sample Project" class="Clust (strict)"("Value"=w942) -> ()  [unwired: 2 in, 2 out]
        n334 = Add(x=w928, y=w929) -> (x+y=w927:T16)
        n335 = Add(x=w933, y=w932) -> (x+y=w931:T16)
        n336 = Add(x=w936, y=w935) -> (x+y=w934:T16)
        n337 = Add(x=w924, y=w925) -> (x+y=w923:T16)
        n338 = Add(x=w921, y=w922) -> (x+y=w920:T16)
        n339 = property on="More Info" class="Str"("Position"=w934) -> ()  [unwired: 2 in, 2 out]
        n340 = property on="More Info" class="Str"("Position"=w931) -> ()  [unwired: 2 in, 2 out]
        n341 = property on="More Info" class="Str"("Position"=w927) -> ()  [unwired: 2 in, 2 out]
        n342 = property on="More Info" class="Str"("Position"=w923) -> ()  [unwired: 2 in, 2 out]
        n343 = property on="More Info" class="Str"("Position"=w920) -> ()  [unwired: 2 in, 2 out]
      }
      frame "Select Available Sample" {
        w963 = T4[] [] items=["Idle", "Initialize", "Parse Config Files", "Update Title", "Update Navigation", "Update Tab", "Load Question", "Load All Samples", "Update Sample Description", "Load Available Samples", "Cancel", "More Information", "Create Project", "Copy Project", "Update Warning", "Update Available Samples", "Select Available Sample", "Load Start Choice", "Show Recommended Sample", "Init Spec Page", "Insert Spec Page", "Stop Spec Page", "Set Control Font", "Focus Previous Selection"]
        # "initialize before draw a new pic"
        n344 = Unbundle By Name(w973) -> ("Selected Sample"=w972:i32, "Scrollbar Value"=w971:i32)
        n345 = Subtract(x=w972, y=w971) -> (x-y=w970:i32)
        n346 = invoke on="Sample Highlight" class="Pict" method="Reinit To Default"(error in=w965) -> (error out=w966:errorcluster)  [unwired: 2 in, 2 out]
        n347 = flat-sequence {
          tunnel: w970 -> [w999]
          tunnel: w966 -> [w985]
          tunnel: [w984] -> w964
          frame #0 {
            w988 = u32 16243333  # Background Color
            w992 = i16 8  # oval width
            n348 = property on="Sample Highlight" class="Pict"() -> ("MasterRect"=w998:T14)  [unwired: 2 in, 2 out]
            n349 = case shown="Default" w999 {
              tunnel: [w1002 w1005 w1008 w1011 w1014 T14 {"Left"=-1000, "Top"=-1000, "Right"=0, "Bottom"=0} ("MasterRect")] -> w995
              tunnel: w985 -> [w1001 w1004 w1007 w1010 w1012 w1015]
              tunnel: [w1000 w1003 w1006 w1009 w1013 w1015] -> w984
              frame 0 {
                n350 = property on="List Item" class="Clust (strict)"(error in=w1001) -> (error out=w1000:errorcluster, "MasterRect"=w1002:T14)  [unwired: 1 in, 1 out]
              }
              frame 1 {
                n351 = property on="List Item 2" class="Clust (strict)"(error in=w1004) -> (error out=w1003:errorcluster, "MasterRect"=w1005:T14)  [unwired: 1 in, 1 out]
              }
              frame 2 {
                n352 = property on="List Item 3" class="Clust (strict)"(error in=w1007) -> (error out=w1006:errorcluster, "MasterRect"=w1008:T14)  [unwired: 1 in, 1 out]
              }
              frame 3 {
                n353 = property on="List Item 4" class="Clust (strict)"(error in=w1010) -> (error out=w1009:errorcluster, "MasterRect"=w1011:T14)  [unwired: 1 in, 1 out]
              }
              frame 4 {
                n354 = property on="List Item 5" class="Clust (strict)"(error in=w1012) -> (error out=w1013:errorcluster, "MasterRect"=w1014:T14)  [unwired: 1 in, 1 out]
              }
              frame Default {
              }
            }
            n355 = Unbundle By Name(w995) -> ("Left"=w980:i16, "Top"=w983:i16)
            n356 = Unbundle By Name(w998) -> ("Left"=w997:i16, "Top"=w996:i16)
            n357 = Subtract(x=w980, y=w997) -> (x-y=w977:i16)
            n358 = Subtract(x=w983, y=w996) -> (x-y=w976:i16)
            n359 = Add(x=w977, y=i16 487) -> (x+y=w978:i16)
            n360 = Add(x=w976, y=i16 60) -> (x+y=w981:i16)
            n361 = Bundle By Name(cluster=w995, "Left"=w977, "Top"=w976, "Right"=w978, "Bottom"=w981) -> (w989:T14)
            n362 = call <vilib>:"Draw Round Rect.vi"("picture"="Sample Highlight", "oval width"=w992, "rect"=w989, "fill?(F)"=TRUE, "color(black)"=w988, "oval height"=w992) -> ("new picture"=w990:picture)  [unwired: 3 in]
            n363 = call <vilib>:"Hilite Color.vi"("Color In"=w988) -> ("Shadow"=w993:u32)  [unwired: 1 in, 1 out]
            n364 = call <vilib>:"Draw Round Rect.vi"("picture"=w990, "oval width"=w992, "rect"=w989, "fill?(F)"=FALSE, "color(black)"=w993, "oval height"=w992) -> ("new picture"=w986:picture)  [unwired: 3 in]
            n365 = property on="Sample Highlight" class="Pict"("Value"=w986) -> ()  [unwired: 2 in, 2 out]
          }
        }
      }
      frame "Load Start Choice" {
        w1022 = FALSE ("Disabled&GrayedOut")
        w1039 = T4[] [] items=["Idle", "Initialize", "Parse Config Files", "Update Title", "Update Navigation", "Update Tab", "Load Question", "Load All Samples", "Update Sample Description", "Load Available Samples", "Cancel", "More Information", "Create Project", "Copy Project", "Update Warning", "Update Available Samples", "Select Available Sample", "Load Start Choice", "Show Recommended Sample", "Init Spec Page", "Insert Spec Page", "Stop Spec Page", "Set Control Font", "Focus Previous Selection"]
        n366 = case shown="\"EL-RIO-CM\"" w1020 {
          selector: w1020 -> [w1051 _]
          tunnel: [w1051 "NI ELVIS RIO Control Module"] -> w1019
          tunnel: ["a" "an"] -> w1018
          frame Default {
          }
          frame "EL-RIO-CM" {
          }
        }
        n367 = property on="Choice 1" class="myRIO Choice Button (strict)"("Disabled&GrayedOut"=w1022) -> (error out=w1025:errorcluster)  [unwired: 2 in, 1 out]
        n368 = property on="Choice 2" class="myRIO Choice Button (strict)"(error in=w1025, "Disabled&GrayedOut"=w1022) -> (error out=w1024:errorcluster)  [unwired: 1 in, 1 out]
        n369 = global read "Wizard Global.vi" "Start Question"() -> (w1017:string)
        n370 = global read "Wizard Global.vi" "Choice1"() -> (w1027:string)
        n371 = Format Into String(format string=w1017, w1018, w1019) -> (resulting string=w1021:string)  [unwired: 2 in, 1 out]
        n372 = property on="Question" class="Str"("Value"=w1021) -> ()  [unwired: 2 in, 2 out]
        n373 = Unbundle By Name(w1044) -> ("Show Guidance"=w1047:bool)
        n374 = global read "Wizard Global.vi" "Choice2"() -> (w1026:string)
        n375 = Pick Line(multi-line string=w1027, line index=0) -> (output string=w1037:string)  [unwired: 1 in]
        n376 = Pick Line(multi-line string=w1027, line index=1) -> (output string=w1036:string)  [unwired: 1 in]
        n377 = property on="Choice 1" class="myRIO Choice Button (strict)"(error in=w1024, "Title"=w1037, "Explanation"=w1036, "Value"=TRUE ("Choice1")) -> (error out=w1023:errorcluster)  [unwired: 1 in, 1 out]
        n378 = Pick Line(multi-line string=w1026, line index=0) -> (output string=w1032:string)  [unwired: 1 in]
        n379 = Pick Line(multi-line string=w1026, line index=1) -> (output string=w1031:string)  [unwired: 1 in]
        n380 = Select(t=Answers."Choice 1" ("Answers"), s=w1047, f=Answers."Choice 2" ("Answers")) -> (s? t:f=w1038:T7)
        n381 = property on="Choice 2" class="myRIO Choice Button (strict)"(error in=w1023, "Title"=w1032, "Explanation"=w1031, "Value"=FALSE ("Choice2")) -> ()  [unwired: 1 in, 2 out]
        n382 = Bundle By Name(cluster=w1044, "Answers"=w1038) -> (w1043:T5)
      }
      frame "Show Recommended Sample" {
        w1056 = T4[] [] items=["Idle", "Initialize", "Parse Config Files", "Update Title", "Update Navigation", "Update Tab", "Load Question", "Load All Samples", "Update Sample Description", "Load Available Samples", "Cancel", "More Information", "Create Project", "Copy Project", "Update Warning", "Update Available Samples", "Select Available Sample", "Load Start Choice", "Show Recommended Sample", "Init Spec Page", "Insert Spec Page", "Stop Spec Page", "Set Control Font", "Focus Previous Selection"]
        n383 = Unbundle By Name(w1066) -> ("Result"=w1062:string)  [unwired: 1 out]
        "Recommended sample" <- w1062
        n384 = Unbundle By Name(w1067) -> ("Item List"=w1065:T9)
        n385 = call "Get Template Page.vi"("Target Name"=w1055, "error in (no error)"=w1058, "Item List"=w1065, "Item Name"=w1062) -> ("error out"=w1057:errorcluster, "Description"=→"Description":string, "picture"=→"Sample Pic 2":picture)  [unwired: 4 in, 1 out]
      }
      frame "Init Spec Page" {
        w1072 = T4[] [] items=["Idle", "Initialize", "Parse Config Files", "Update Title", "Update Navigation", "Update Tab", "Load Question", "Load All Samples", "Update Sample Description", "Load Available Samples", "Cancel", "More Information", "Create Project", "Copy Project", "Update Warning", "Update Available Samples", "Select Available Sample", "Load Start Choice", "Show Recommended Sample", "Init Spec Page", "Insert Spec Page", "Stop Spec Page", "Set Control Font", "Focus Previous Selection"]
        n386 = call <resource>:"Parse Category Overrides.vi"() -> ("Non Localized Names"=w1092:string[], "Names"=w1091:string[])  [unwired: 9 in, 1 out]
        n387 = call <resource>:"GetAllTemplates.vi"("Category Nonlocalized Names"=w1092, "Category Names"=w1091) -> ("Templates Out"=w1086:refnum<class "MetaDataObj.lvclass">[])  [unwired: 9 in]
        n388 = call-by-ref "?"(error in=w1074, "key"=w1082) -> ("error out"=w1069:errorcluster, "found?"=w1088:bool, "value"=w1087:path[])  [unwired: 5 in, 2 out]
        n389 = Empty Array?(array=w1087) -> (empty?=w1089:bool)
        n390 = for {
          tunnel: w1086 -> [w1102] mode=indexing
          tunnel: [w1099] -> w1079
          tunnel: w1077 -> [w1098]
          shift-right: [w1096] -> w1070
          shift-left: w1074 -> [w1097]
          stop <- w1100 stop-if-true
          n391 = property class="MetaDataObj.lvclass"(reference=w1102, error in=w1097) -> (reference out=w1099:refnum<class "MetaDataObj.lvclass">, error out=w1096:errorcluster, "Title"=w1101:string)
          n392 = Equal?(x=w1101, y=w1098) -> (x = y?=w1100:bool)
        }
        n393 = Compound Arithmetic op=AND(invert w1089, w1088) -> (w1090:bool)
        n394 = case shown="False" w1090 {
          tunnel: w1087 -> [_ w1106]
          tunnel: [w1103 w1104] -> w1080
          frame False {
            n395 = call <vilib>:"Dflt Data Dir.vi"() -> ("App:Default Data Directory"=w1103:path)
          }
          frame True {
            n396 = Index Array(array=w1106) -> (element=w1105:path)  [unwired: 1 in]
            n397 = Strip Path(path=w1105) -> (stripped path=w1104:path)  [unwired: 1 out]
          }
        }
        n398 = Merge Errors(w1070, w1069) -> (w1071:errorcluster)
        n399 = call "Load Sample Custom VI.vi"("error in"=w1071, "Title"=w1077, "Template"=w1079) -> ("error out"=w1076:errorcluster, "Template out"=w1078:refnum<class "MetaDataObj.lvclass">)  [unwired: 6 in, 1 out]
        n400 = property class="MetaDataObj.lvclass"(reference=w1078, error in=w1076, "Project Root"=w1080) -> (reference out=w1085:refnum<class "MetaDataObj.lvclass">, error out=w1075:errorcluster)
        n401 = call-by-ref "?"(error in=w1075, "MetaDataObj in"=w1085) -> (error out=w1073:errorcluster, "MetaDataObj out"=w1084:refnum<class "MetaDataObj.lvclass">)  [unwired: 11 in, 1 out]
      }
      frame "Insert Spec Page" {
        w1107 = T4[] [] items=["Idle", "Initialize", "Parse Config Files", "Update Title", "Update Navigation", "Update Tab", "Load Question", "Load All Samples", "Update Sample Description", "Load Available Samples", "Cancel", "More Information", "Create Project", "Copy Project", "Update Warning", "Update Available Samples", "Select Available Sample", "Load Start Choice", "Show Recommended Sample", "Init Spec Page", "Insert Spec Page", "Stop Spec Page", "Set Control Font", "Focus Previous Selection"]
        w1141 = refnum<user-event> refnum  # Null Event
        w1142 = T17 {"\"Tab Forward To\" Refnum"=refnum, "\"Tab Backward To\" Refnum"=refnum, "Errors"=refnum, "Quit"=refnum}  # Wizard Interface
        n402 = Unbundle By Name(w1130) -> ("Result"=w1132:string, "Show Guidance"=w1131:bool, "Selected Sample"=w1128:i32)
        n403 = Unbundle By Name(w1129) -> ("Sample Item Names"=w1133:string[], "Item List"=w1126:T9)
        n404 = call-dynamic "Fire Quit Event.vi"("Force Quit?"=TRUE, "BaseSpecPage in"=w1118) -> ()  [unwired: 7 in, 3 out]
        n405 = control-ref of="This VI"() -> (w1120:refnum<vi>)
        n406 = Bundle(cluster=w1142, "\"Tab Forward To\" Refnum"=w1140, "\"Tab Backward To\" Refnum"=w1139, "Errors"=w1138, "Quit"=w1141) -> (w1137:T17)
        n407 = case shown="False" w1131 {
          tunnel: [w1146 w1147] -> w1127
          tunnel: w1133 -> [w1145 _]
          tunnel: w1132 -> [_ w1147]
          tunnel: w1128 -> [w1144 _]
          frame False {
            n408 = Index Array(array=w1145, index=w1144) -> (element=w1146:string)
          }
          frame True {
          }
        }
        n409 = call-by-ref "?"(error in=w1124, "Defer?"=TRUE ("Visible"), "VI in"=w1120) -> ("error out"=w1113:errorcluster)  [unwired: 10 in, 2 out]
        n410 = call "Find Item By Tag.vi"("Tag"=w1127, "Item List"=w1126) -> ("Item Info"=w1116:T10)  [unwired: 9 in]
        n411 = call "Update Sample Meta Data.vi"("error in"=w1113, "Item Info"=w1116, "MetaDataObj"=w1115) -> ("error out"=w1112:errorcluster, "MetaDataObj out"=w1114:refnum<class "MetaDataObj.lvclass">)  [unwired: 7 in]
        n412 = call-by-ref "?"(error in=w1112, "Wizard Interface"=w1137, "MetaDataObj"=w1114) -> (error out=w1110:errorcluster, "VI Ref Out"=w1109:refnum<vi>, "SpecPage out"=w1117:refnum<class "BaseSpecPage.lvclass">, "SpecPage Ctrl #n Ref"=w1111:refnum<vi>, "SpecPage Ctrl #1 Ref"=w1135:refnum<vi>)  [unwired: 7 in, 1 out]
        n413 = Bundle By Name(cluster=w1129, "Spec Page Reference"=w1109, "CurPage Ctrl #n"=w1111, "CurPage Ctrl #1"=w1135) -> (w1136:T8)
        n414 = invoke class="VI" method="FP.Close"(reference=w1109) -> (reference out=w1108:refnum<vi>)  [unwired: 2 in, 2 out]
        n415 = invoke on="Spec Page" class="SubPanel" method="Insert VI"(error in=w1110, "VI Ref"=w1108) -> (error out=w1122:errorcluster)  [unwired: 2 in, 3 out]
        n416 = call-by-ref "?"(error in=w1122, "Defer?"=FALSE ("Visible"), "VI in"=w1120) -> ("error out"=w1121:errorcluster)  [unwired: 10 in, 2 out]
      }
      frame "Stop Spec Page" {
        w1148 = T4[] [] items=["Idle", "Initialize", "Parse Config Files", "Update Title", "Update Navigation", "Update Tab", "Load Question", "Load All Samples", "Update Sample Description", "Load Available Samples", "Cancel", "More Information", "Create Project", "Copy Project", "Update Warning", "Update Available Samples", "Select Available Sample", "Load Start Choice", "Show Recommended Sample", "Init Spec Page", "Insert Spec Page", "Stop Spec Page", "Set Control Font", "Focus Previous Selection"]
        # "Sync the updates of Subpanel to its MetaDataObj"
        n417 = call-dynamic "Fire Quit Event.vi"("error in (no error)"=w1154, "BaseSpecPage in"=w1152) -> ("error out"=w1158:errorcluster, "Quit OK?"=w1150:bool, "BaseSpecPage out"=w1157:refnum<class "BaseSpecPage.lvclass">)  [unwired: 7 in]
        n418 = case shown="True" w1150 {
          tunnel: w1157 -> [w1164 w1169]
          tunnel: w1158 -> [w1163 w1168]
          tunnel: [w1164 refnum<class "BaseSpecPage.lvclass"> refnum ("BaseSpecPage out")] -> w1151
          tunnel: [w1163 w1166] -> w1153
          tunnel: [w1162 w1165] -> w1155
          tunnel: w1156 -> [w1162 _]
          frame False {
          }
          frame True {
            n419 = call-dynamic "Finalize.vi"("error in (no error)"=w1168, "BaseSpecPage in"=w1169) -> ("error out"=w1166:errorcluster, "MetaDataObj out"=w1165:refnum<class "MetaDataObj.lvclass">)  [unwired: 7 in, 1 out]
          }
        }
      }
    }
    n420 = case shown="Error" w67 {
      selector: w67 -> [w91 w99]
      tunnel: w66 -> [w90 _]
      tunnel: [w91 w106] -> w65
      tunnel: [w90 w102] -> w64
      tunnel: w63 -> [w89 w104]
      tunnel: [w89 w105] -> w62
      tunnel: w53 -> [_ w92]
      frame No Error {
      }
      frame Error {
        w102 = T4[] [] items=["Idle", "Initialize", "Parse Config Files", "Update Title", "Update Navigation", "Update Tab", "Load Question", "Load All Samples", "Update Sample Description", "Load Available Samples", "Cancel", "More Information", "Create Project", "Copy Project", "Update Warning", "Update Available Samples", "Select Available Sample", "Load Start Choice", "Show Recommended Sample", "Init Spec Page", "Insert Spec Page", "Stop Spec Page", "Set Control Font", "Focus Previous Selection"]
        n421 = global read "Wizard Global.vi" "Error dialog"() -> (w94:string)
        n422 = Unbundle By Name(w99) -> ("code"=w97:i32, "source"=w96:string)
        n423 = Flush Queue(queue=w104) -> (queue out=w101:refnum<queue>, error out=w100:errorcluster)  [unwired: 1 in, 1 out]
        n424 = Format Into String(format string=w94, w92) -> (resulting string=w93:string)  [unwired: 2 in, 1 out]
        n425 = Format Into String(format string="Error code: %d\\nError source: %s\\n %s", w97, w96, w93) -> (resulting string=w95:string)  [unwired: 2 in, 1 out]
        n426 = Enqueue Element(queue=w101, element=States."Cancel", error in (no error)=w100) -> (queue out=w105:refnum<queue>, error out=w106:errorcluster)  [unwired: 1 in, 1 out]
        n427 = One Button Dialog(message=w95) -> ()  [unwired: 1 in, 1 out]
      }
    }
    n428 = for {
      tunnel: w64 -> [w107] mode=indexing
      shift-right: [w111] -> w84
      shift-left: w62 -> [w108]
      shift-right: [w110] -> w81
      shift-left: w65 -> [w109]
      n429 = Enqueue Element(queue=w108, element=w107, error in (no error)=w109) -> (queue out=w111:refnum<queue>, error out=w110:errorcluster)  [unwired: 1 in, 1 out]
    }
  }
  n430 = Flush Queue(queue=w24, error in (no error)=w21) -> (queue out=w23:refnum<queue>, error out=w22:errorcluster)  [unwired: 1 out]
  n431 = Release Queue(queue=w23, error in (no error)=w22) -> (error out=w30:errorcluster)  [unwired: 1 in, 2 out]
  n432 = Unregister For Events(event registration refnum=w31, error in=w30) -> (error out=w32:errorcluster)
  n433 = Destroy User Event(user event=w5, error in=w32) -> (error out=w7:errorcluster)
  n434 = Destroy User Event(user event=w6, error in=w7) -> (error out=w4:errorcluster)
  n435 = invoke class="VI" method="FP.Close"(error in=w4) -> ()  [unwired: 2 in, 3 out]
